vi "9_3_1_2 No_Load_Test_Set 12V for PS1-PS3.vi"(11 "VariantIn":variant caption="Test Config Cluster Variant In") -> (0 "System Error Out":errorcluster, 3 "variantOut":variant caption="Test Config Cluster V ariant Out")   [LabVIEW 2020]
uses:
  <vilib>/Utility/miscctls.llb/LVRowAndColumnTypeDef.ctl
  <userlib>/_ATMF/Tools/Control/__TEST__SEQ__VARIABLES__.ctl
  <userlib>/_ATMF/Tools/Control/__STEP__DATA__.ctl
  <userlib>/_ATMF/Tools/Control/__STEP__DATA__TYPE__.ctl
  <userlib>/_ATMF/Tools/Control/__STEP__DATA__STATUS__TYPE__.ctl
  <userlib>/_ATMF/Tools/Control/__TEST__SEQ__CONFIG__CLUSTER__.ctl
  <userlib>/_ATMF/Control_Typedef/__TEST__STEP__VAR__UI__EXEC__MODE__.ctl
  <vilib>/Utility/miscctls.llb/LVBoundsTypeDef.ctl
  <vilib>/Utility/miscctls.llb/LVPositionTypeDef.ctl
  <userlib>/_ATMF/Tools/Control/__TABLE__ACTION__.ctl
  subvi/DM3058 Function Choose.ctl
  subvi/DCDC_Command.ctl
  70cdd13f-c836-49cb-97c4-706e2b611909.vi
  367b9f9e-7b96-452b-b4ff-c6404e92ffb7.vi
  <vilib>/Utility/file.llb/Write Delimited Spreadsheet (string).vi
  <vilib>/Utility/file.llb/Read Delimited Spreadsheet (string).vi
  <userlib>/_ATMF/Tools/SubVIs/SubPalette_Update_Sequencer_Variable/SEQ.Update_Seq_Var_Module.Action.vi
  <userlib>/_ATMF/Tools/SubVIs/SubPalette_Update_Sequencer_Variable/Set_Max_Min/SEQ.Update_Seq_Var_Module.Set_Max_Min.vi
  <userlib>/_ATMF/Tools/SubVIs/SubPalette_Update_Sequencer_Variable/SEQ.Update_Seq_Var_Module.Numericl_Test.vi
  <userlib>/_ATMF/Tools/SubVIs/SubPalette_Update_Sequencer_Variable/SEQ.Update_Seq_Var_Module.Pass_Fail_Test.vi
  <vilib>/Comparison/Equal/Equal Functor/Equal Functor.lvclass
  <vilib>/addons/_JKI.lib/Serialization/JSON/JKI JSON Serialization.lvlib
panel:
  in  "Instrument Serial":T1
  out "Cell Position":T2
  in  "stepsRing":u16(ring) items=["Next", "End", "--------------", "init", "Power On", "Measure VPS1", "Measure VPS2", "Measure VPS3", "Measure L1 ON", "Measure L3 ON", "Measure UUT D3 ON", "Measure UUT D5 ON", "Measure UUT D6 ON", "Measure UUT D8 ON", "Measure APOS UUT Voltages", "Measure ANEG UUT Voltages", "Measure DPOS UUT Voltages"]
  in  "exitButton":bool
  in  "saveButton":bool
  in  "runButton":bool
  in  "currentRetest":u8
  in  "totalSeqIndex":i32
  in  "currenIndex":i32
  in  "seqData[](Process)":string[][](array[string])
  in  "disMsg":refnum<vi>
  in  "seqData[](Original)":string[][](array[string])
  in  "Tab Control":enum32{"Sequence", "Input", "Output"}(tab)
  in  "stepName":string
  in  "Sequence List":i32[](listbox)=[0]
  in  "seqFilePath":path caption="Sequence File Path :"
  in  "userDef":T3={"VSP1 Min"=13.0, "VSP1 Max"=11.0, "VSP2 Min"=13.0, "VSP3 Max"=11.0, "VSP3 Min"=13.0, "VSP2 Max"=11.0, "L1 Min"=1.164, "L1 Max"=1.236, "L3 Min"=1.164, "L3 Max"=1.236, "APOS Max "=0.5, "ANEG Max"=-0.5, "DPOS Max"=0.5, "D5 Min"=1.164, "D5 Max"=1.236, "D6 Min"=1.164, "D6 Max"=1.236, "D3 Min"=0.873, "D3 Max"=0.927, "D8 Min"=1.164, "D8 Max"=1.236, "APOS Min"=0.5, "ANEG Min"=-0.5, "DPOS Min"=0.5} caption="User Input ( Save by Run Ctrl+R and click \"Save\" button  )"
  in  "varFilePath":path caption="Variable File Path :"
  in  "criteriaINI":path caption="Criteria(.ini) Path :"
  in  "displayMsg":string caption="Display Message"
  in  "testTable":i32(listbox)=-1 caption="Connectivity Test"
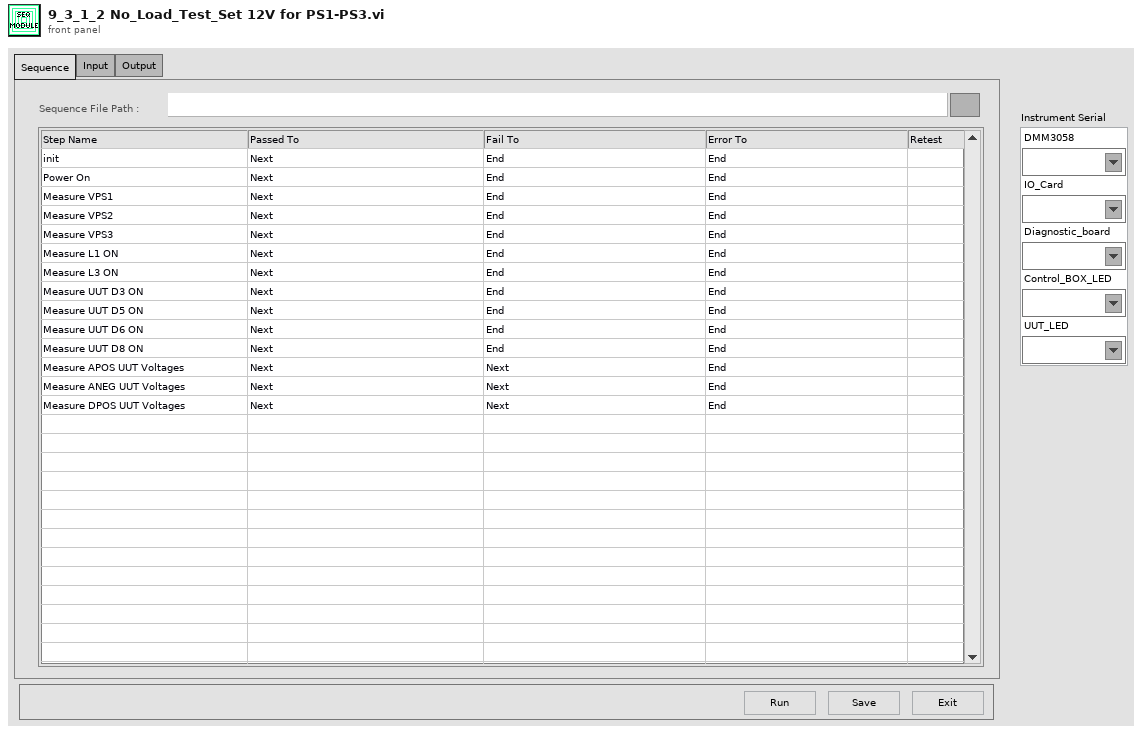
[diagram p1: front panel]
types:
  T1 = cluster{"DMM3058":refnum<visa-resource-name>, "IO_Card":refnum<visa-resource-name>, "Diagnostic_board":refnum<visa-resource-name>, "Control_BOX_LED":refnum<visa-resource-name>, "UUT_LED":refnum<visa-resource-name>}
  T2 = typedef "LVRowAndColumnTypeDef.ctl" = cluster{"Row":i32, "Column":i32}
  T3 = cluster{"VSP1 Min":dbl, "VSP1 Max":dbl, "VSP2 Min":dbl, "VSP3 Max":dbl, "VSP3 Min":dbl, "VSP2 Max":dbl, "L1 Min":dbl, "L1 Max":dbl, "L3 Min":dbl, "L3 Max":dbl, "APOS Max ":dbl, "ANEG Max":dbl, "DPOS Max":dbl, "D5 Min":dbl, "D5 Max":dbl, "D6 Min":dbl, "D6 Max":dbl, "D3 Min":dbl, "D3 Max":dbl, "D8 Min":dbl, "D8 Max":dbl, "APOS Min":dbl, "ANEG Min":dbl, "DPOS Min":dbl}
  T4 = typedef "__TEST__SEQ__VARIABLES__.ctl" = cluster{"stepData":T5, "testConfigCluster":T8}
  T5 = typedef "__STEP__DATA__.ctl" = cluster{"stepType":T6, "stepName":string, "description":string, "min":string, "measure":string, "max":string, "unit":string, "statusType":T7, "runMode":enum16{"Normal", "Skip"}, "viPath":path, "uutError":errorcluster, "passTo":string, "failTo":string, "errorTo":string, "parameter":string, "value":variant, "startTime":timestamp, "intervalLoop":u8, "retest":u8}
  T6 = typedef "__STEP__DATA__TYPE__.ctl" = enum16{"Action", "Pass/Fail Test", "Numeric Limit Test", "String Value Test"}
  T7 = typedef "__STEP__DATA__STATUS__TYPE__.ctl" = enum16{"DONE", "PASS", "FAIL", "ERROR", "SKIPPED"}
  T8 = typedef "__TEST__SEQ__CONFIG__CLUSTER__.ctl" = cluster{"slotIndex":u8, "execMode":T9, "mainConfigFile":path, "criteriaINI":path, "totalResult":bool, "stopIfFail":bool, "userControls":cluster{"dialog":refnum<vi>, "testTable":refnum<vi>, "stopButton":refnum<vi>, "statusBox":refnum<vi>}, "testedResult":enum16{"DONE", "PASS", "FAIL", "ERROR", "SKIPPED"}, "timeStamp":cluster{"Start":timestamp, "End":timestamp}, "repeatNum":u8, "uutInfo":cluster{"s/n":string, "p/n":string, "productRev":string}, "sysLanguage":enum16{"English", "Chinese", "Thai"}, "numOfSocket#":u8, "testRef":string, "testInfo":cluster{"testTime":string, "userID":string, "stationName":string, "testerID":string, "hwVer":string, "swVer":string, "fixtureID":string}}
  T9 = typedef "__TEST__STEP__VAR__UI__EXEC__MODE__.ctl" = enum16{"Run", "Debug", "Edit", "Open VI"}
  T10 = enum16{"open", "replace", "create", "open or create", "replace or create", "replace or create with confirmation"}
  T11 = typedef "LVPositionTypeDef.ctl" = cluster{"Left":i32, "Top":i32}
  T12 = typedef "LVBoundsTypeDef.ctl" = cluster{"Width":u32, "Height":u32}
  T13 = enum32{"Bad", "Idle", "Run top level", "Running"}
  T14 = typedef "__TABLE__ACTION__.ctl" = enum16{"Initial", "Append", "Clear", "Header"}
  T15 = enum16{"StepName", "PassTo", "FailTo", "ErrorTo", "Re-test"}
  T16 = enum16{"StepName", "PassTo", "FailTo", "ErrorTo"}
  T17 = cluster{"Reset (True)":bool, "ID Query (True)":bool, "Auto Range (T:Enable)":bool, "Function (0: DC Volts)":u16, "Range Select":enum16{"200mV", "2V", "20V", "200V", "1000V"}, "Absolute Resolution (0: 5.5 Rate:Slow)":u16}
  T18 = typedef "DM3058 Function Choose.ctl" = enum16{"Close", "Measure", "Config", "Init"}
  T19 = typedef "DCDC_Command.ctl" = enum16{"Reset", "APOS_SENSE", "ANEG_SENSE", "DPOS_SENSE", "FCT_SW1", "FCT_SW2", "FCT_SW3", "ANEG_LOAD", "APOS_LOAD", "DPOS_LOAD", "Short ANEG", "Short APOS", "Short DPOS", "meas_PSU_1_12V", "meas_PSU_2_12V", "meas_PSU_3_12V", "meas_UUT_APOS_voltage", "meas_UUT_ANEG_voltage", "meas_UUT_DPOS_voltage", "meas_LOAD_APOS_voltage", "meas_LOAD_ANEG_voltage", "meas_LOAD_DPOS_voltage", "UUT_FCT_power_SW", "Burn_in_FAN_SW", "FCT_FAN_SW", "FCT_24V_SW", "USB_Reset", "DMM_SW"}
  T20 = typedef "LVPoint32TypeDef.ctl" = cluster{"Horizontal":i32, "Vertical":i32}
  T21 = typedef "LVFontTypeDef.ctl" = cluster{"Font Name":string, "Size":u16, "Bold":bool, "Italic":bool, "Underline":bool, "Strikeout":bool, "Color":u32}
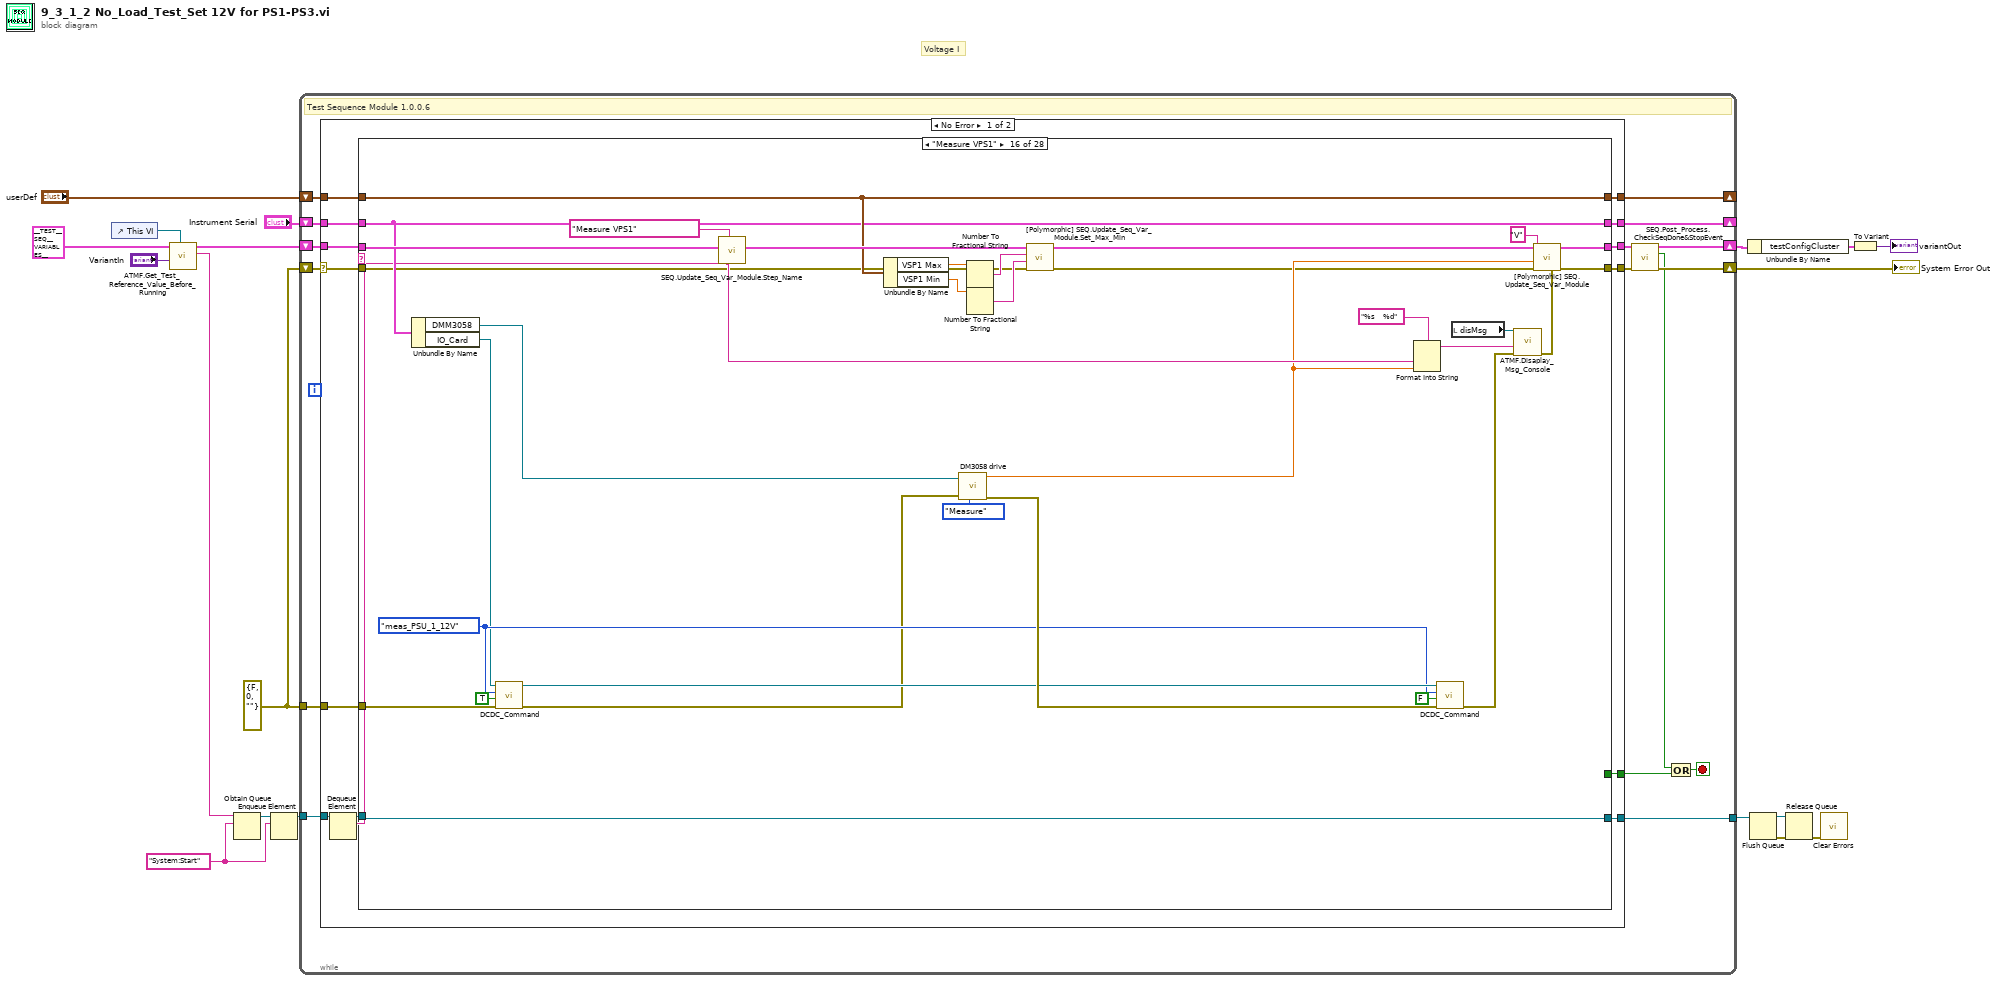
[diagram p0: block diagram]
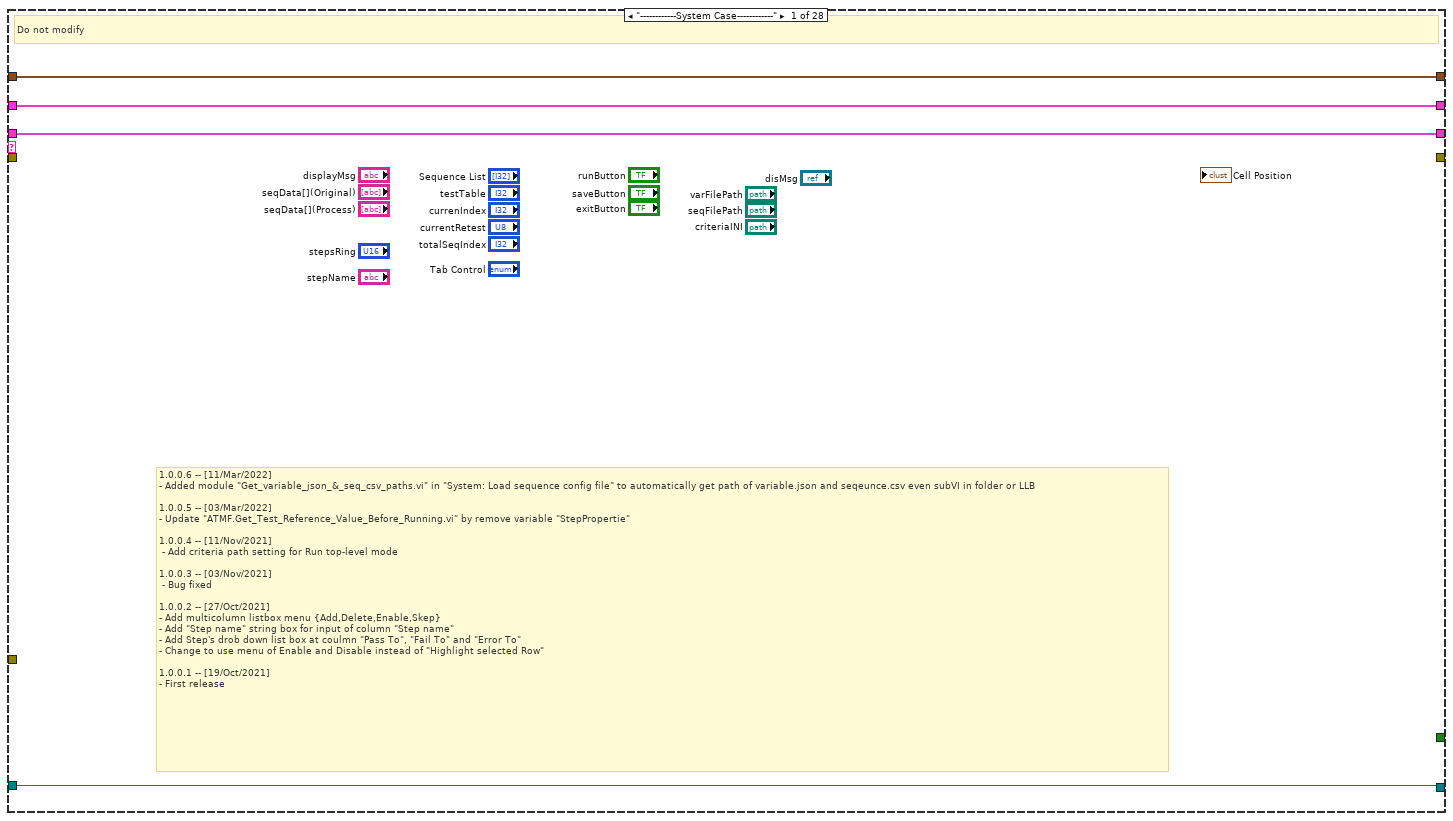
[diagram p2: hidden frame]
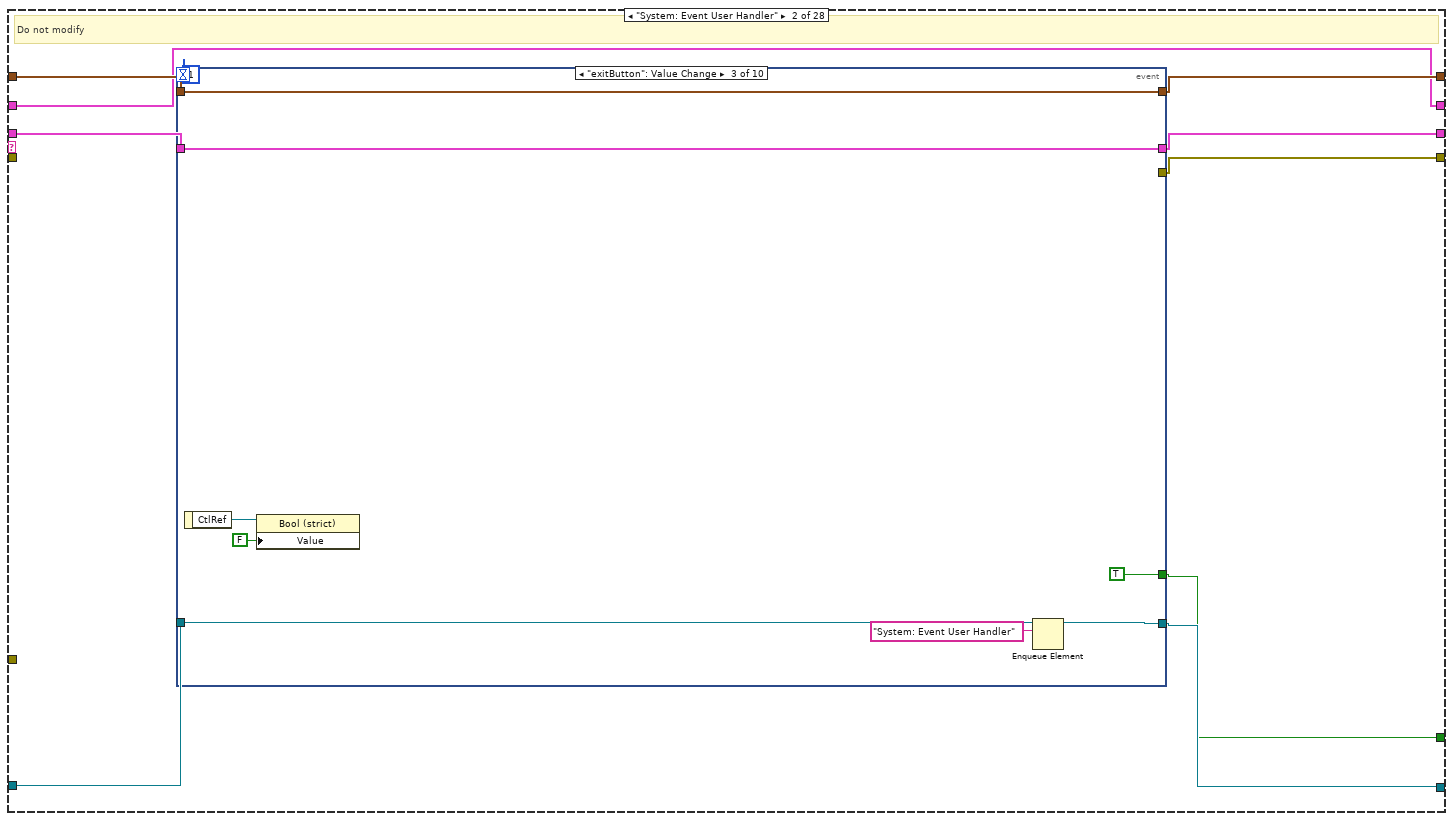
[diagram p3: hidden frame]
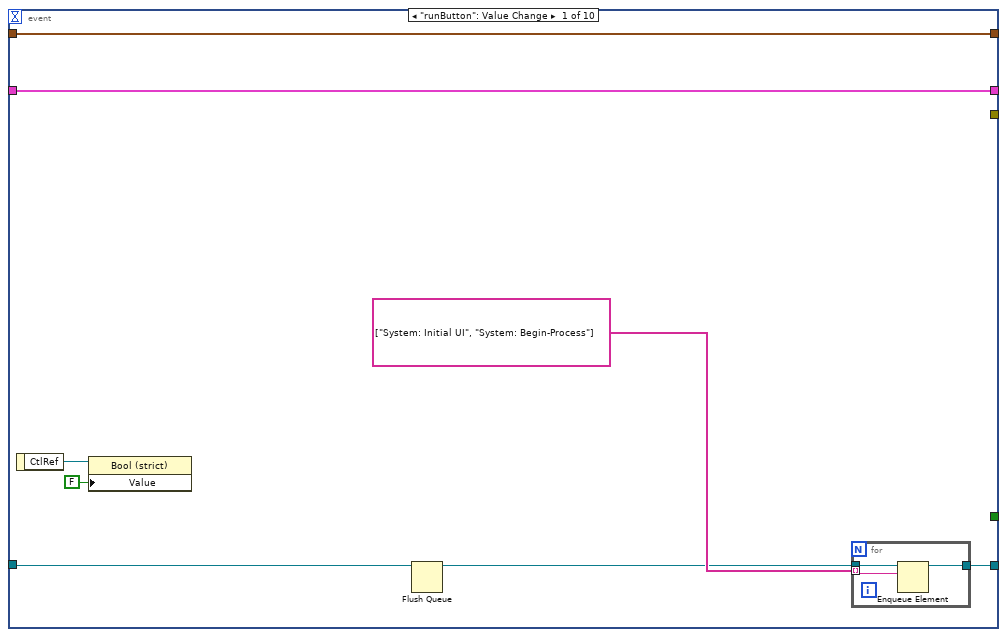
[diagram p4: hidden frame]
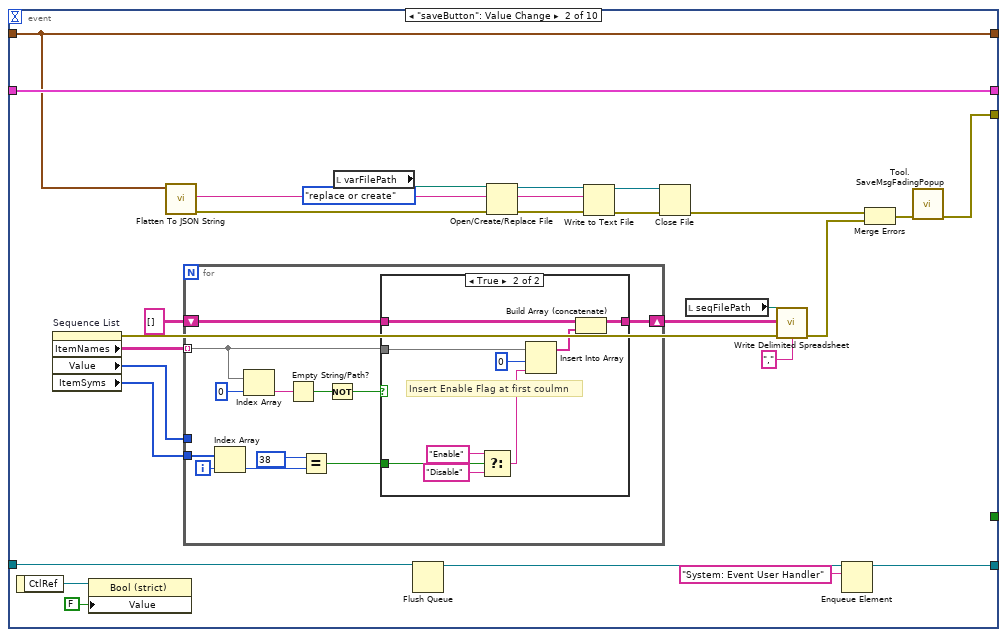
[diagram p5: hidden frame]
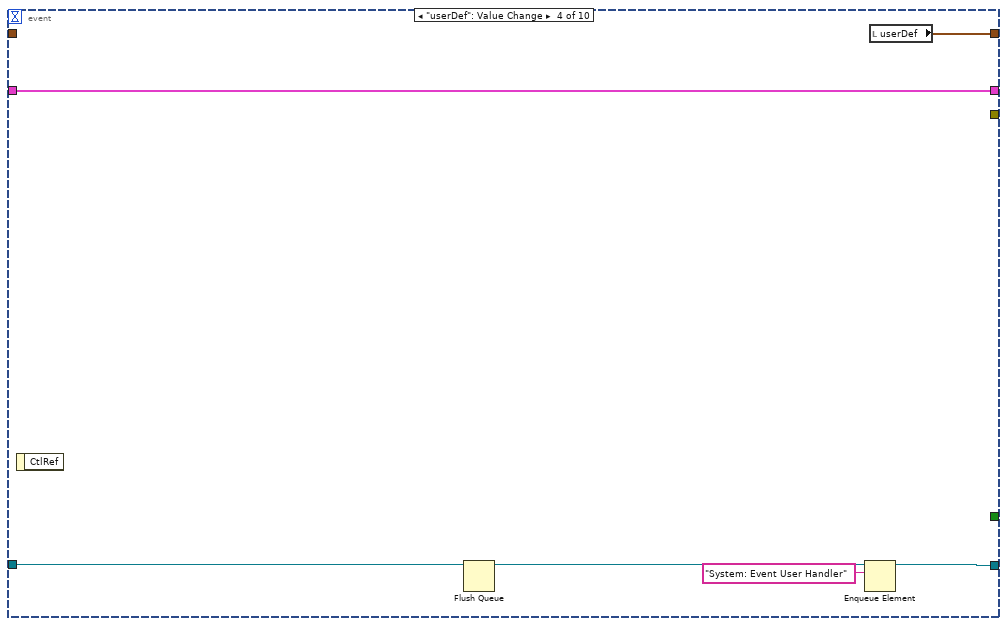
[diagram p7: hidden frame]
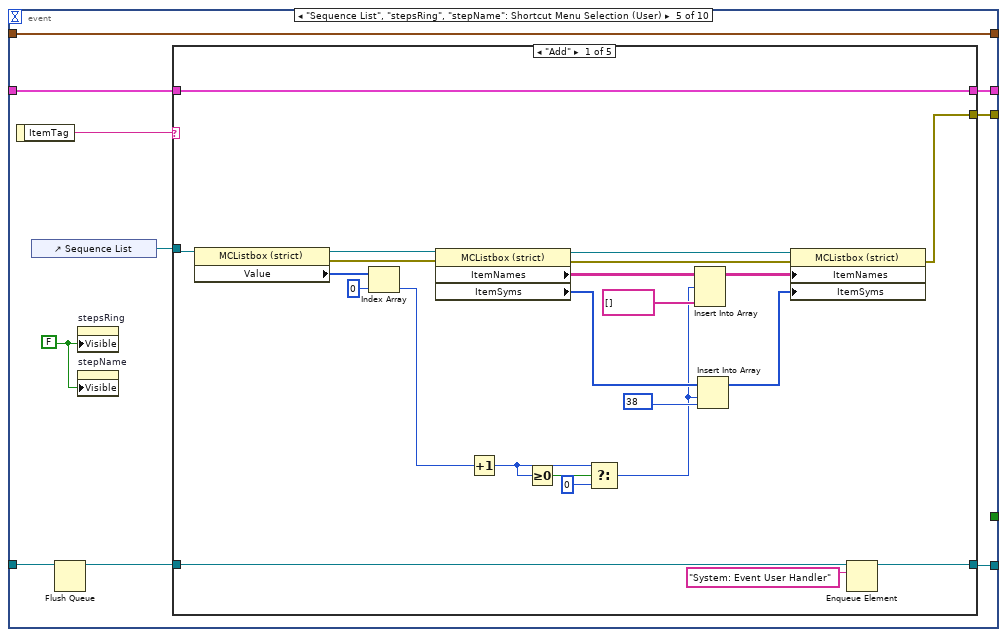
[diagram p8: hidden frame]
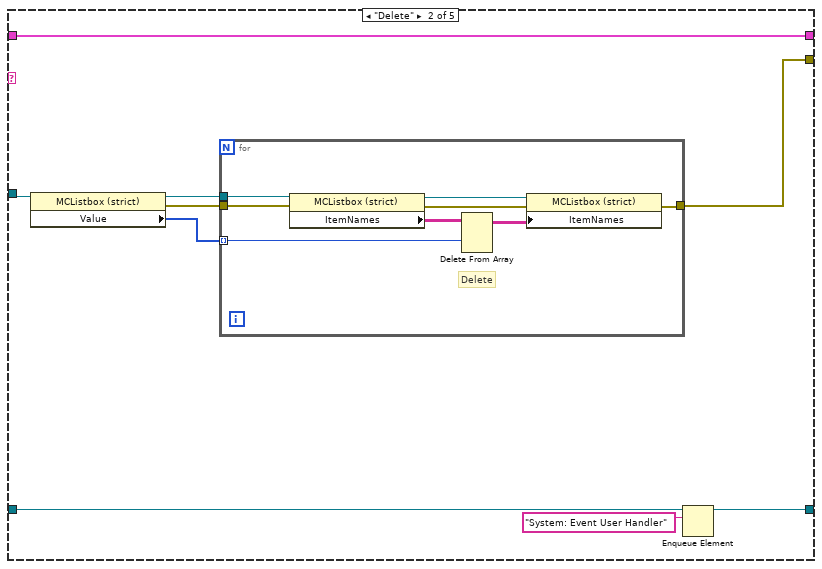
[diagram p9: hidden frame]
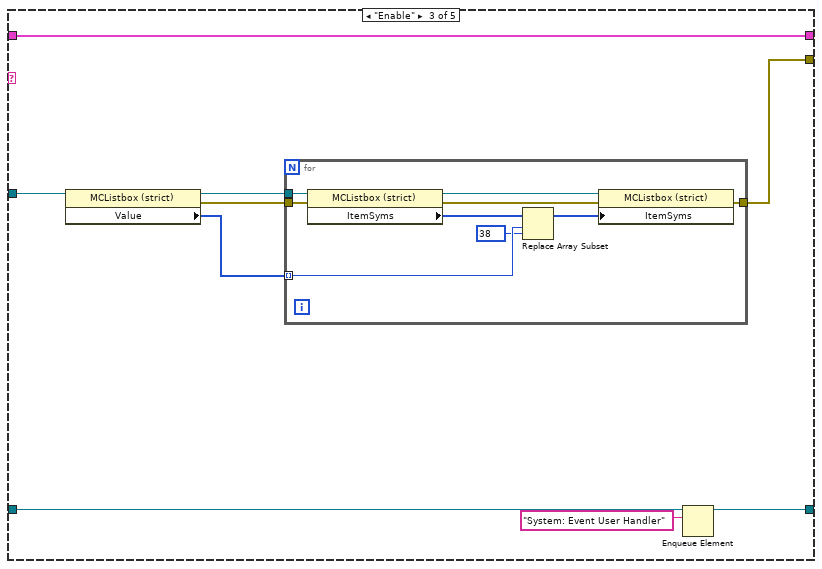
[diagram p10: hidden frame]
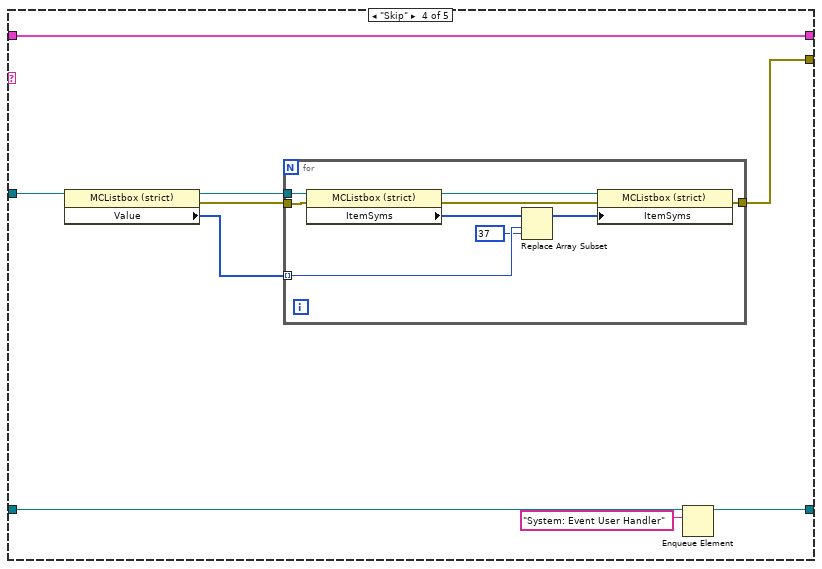
[diagram p11: hidden frame]
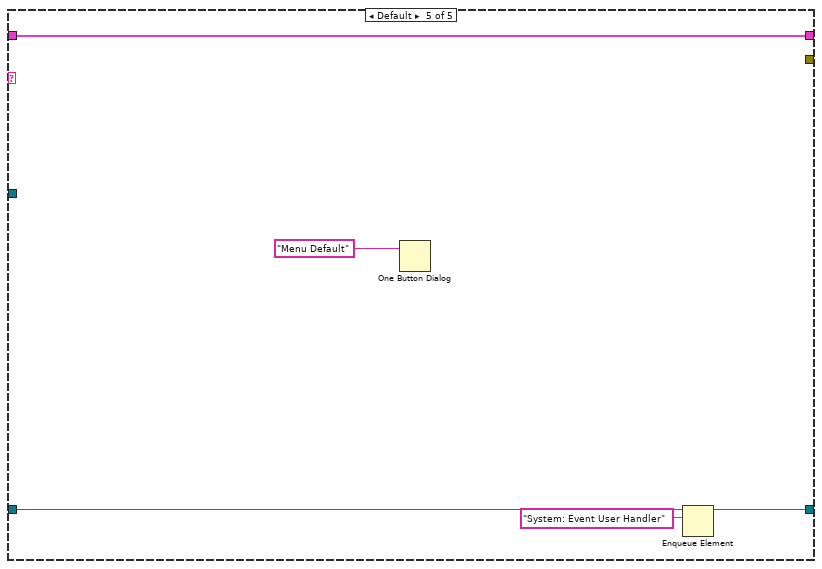
[diagram p12: hidden frame]
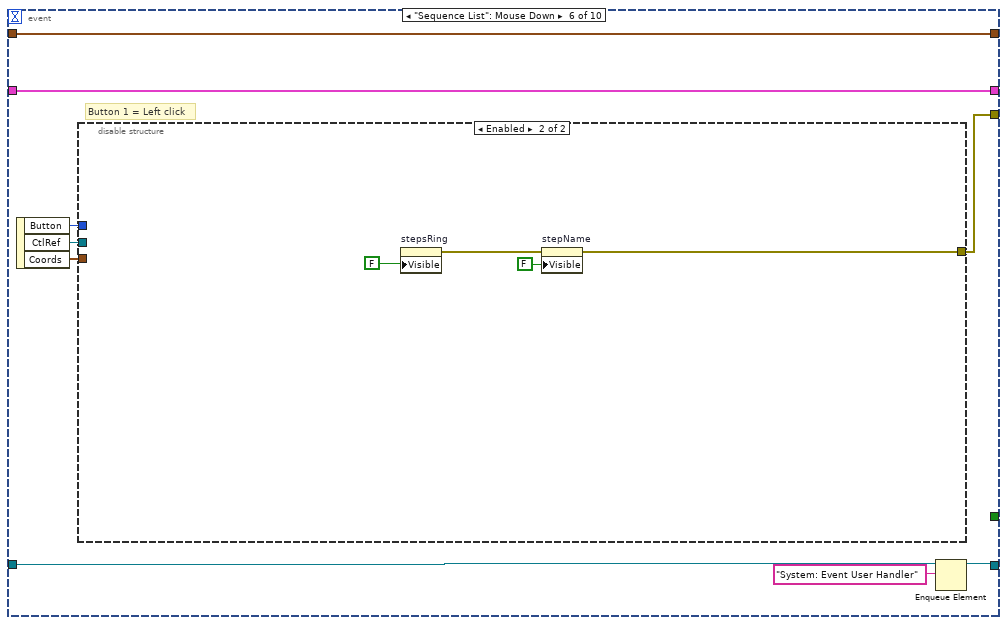
[diagram p13: hidden frame]
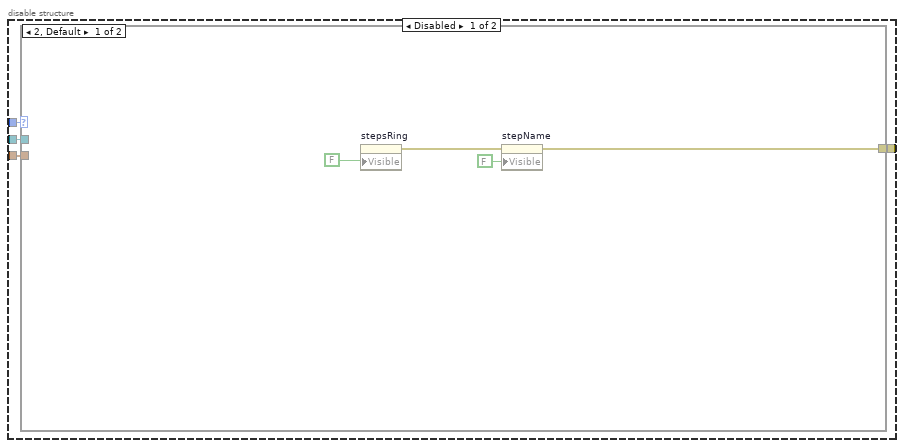
[diagram p14: hidden frame]
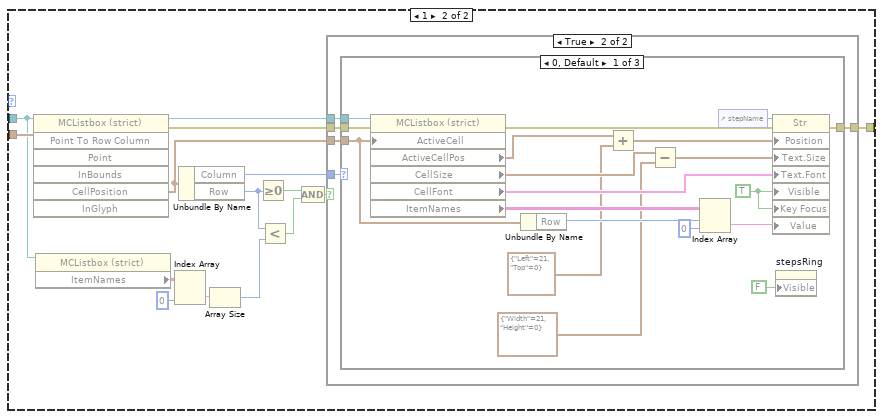
[diagram p15: hidden frame]
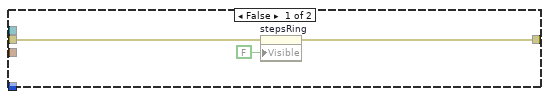
[diagram p16: hidden frame]
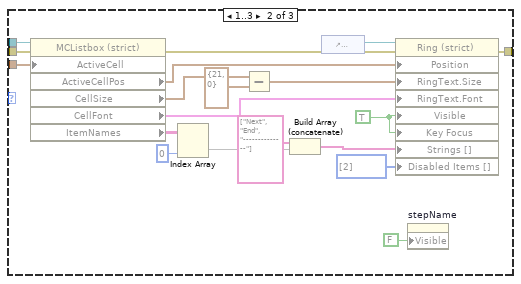
[diagram p17: hidden frame]
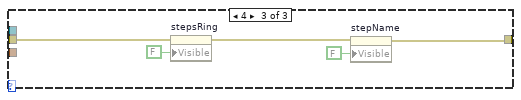
[diagram p18: hidden frame]
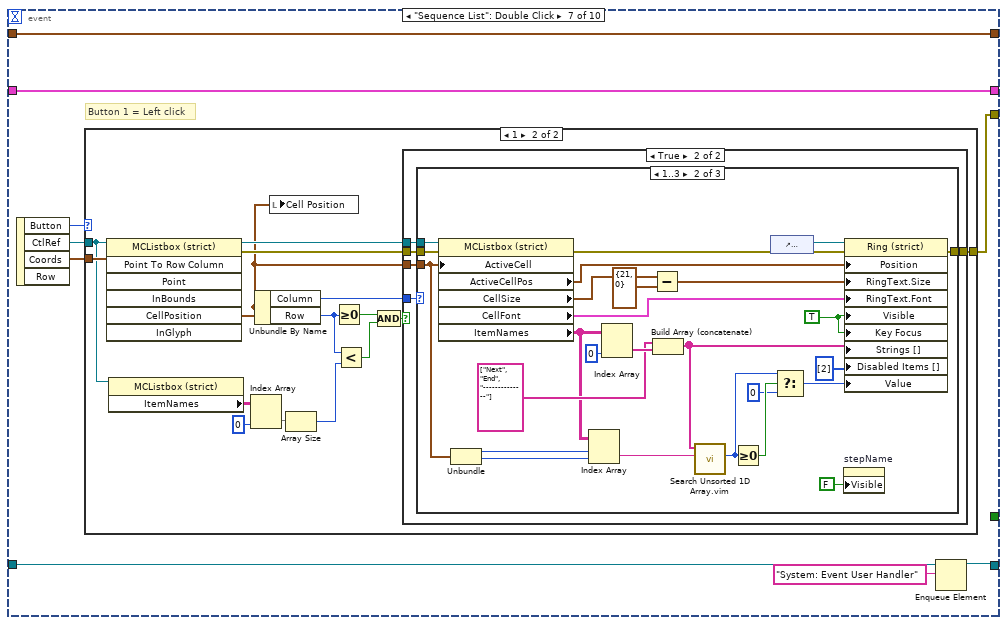
[diagram p19: hidden frame]
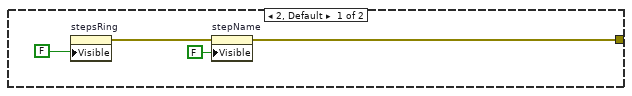
[diagram p20: hidden frame]
diagram:
  w2 = errorcluster {"status"=FALSE, "code"=0, "source"=""} ("UUT Error In")
  w14 = "System:Start"
  # "Voltage I"
  n1 = control-ref of="This VI"() -> (w6:refnum<vi>)
  n2 = call <userlib>:"ATMF.Get_Test_Reference_Value_Before_Running.vi"("viRef"=w6, "Variant"="VariantIn", "seqDataIn"=T4 {"stepData"={"stepType"=enum."Action", "stepName"="", "description"="", "min"="", "measure"="", "max"="", "unit"="", "statusType"=enum."DONE", "runMode"=enum."Normal", "viPath"=path "", "uutError"={"status"=FALSE, "code"=0, "source"=""}, "passTo"="", "failTo"="", "errorTo"="", "parameter"="", "value"=variant(string[][] []), "startTime"=timestamp(0 s since 1904-01-01), "intervalLoop"=1, "retest"=0}, "testConfigCluster"={"slotIndex"=0, "execMode"=enum."Run", "mainConfigFile"=path "", "criteriaINI"=path "", "totalResult"=FALSE, "stopIfFail"=FALSE, "userControls"={"dialog"=refnum, "testTable"=refnum, "stopButton"=refnum, "statusBox"=refnum}, "testedResult"=enum."DONE", "timeStamp"={"Start"=timestamp(0 s since 1904-01-01), "End"=timestamp(0 s since 1904-01-01)}, "repeatNum"=1, "uutInfo"={"s/n"="", "p/n"="", "productRev"=""}, "sysLanguage"=enum."English", "numOfSocket#"=1, "testRef"="", "testInfo"={"testTime"="", "userID"="", "stationName"="", "testerID"="", "hwVer"="", "swVer"="", "fixtureID"=""}}} ("localVar")) -> ("testRef#"=w9:string, "seqDataOut"=w7:T4)  [unwired: 6 in, 1 out]
  n3 = Obtain Queue(name (unnamed)=w9, element data type=w14) -> (queue out=w19:refnum<queue>)  [unwired: 3 in, 2 out]
  n4 = Enqueue Element(queue=w19, element=w14) -> (queue out=w17:refnum<queue>)  [unwired: 2 in, 2 out]
  n5 = while {
    shift-right: [w25] -> w11
    shift-left: w2 -> [w35]
    shift-right: [w27] -> w5
    shift-left: w7 -> [w34]
    tunnel: w17 -> [w33]
    tunnel: [w32] -> w16
    tunnel: w2 -> [w30]
    shift-right: [w29] -> _
    shift-left: "userDef" -> [w31]
    shift-right: [w21] -> _
    shift-left: "Instrument Serial" -> [w20]
    stop <- w22 stop-if-true
    # "Test Sequence Module 1.0.0.6"
    n6 = case shown="No Error" w35 {
      selector: w35 -> [w47 w1245]
      tunnel: [w46 w1245] -> w26
      tunnel: w34 -> [w49 w1252]
      tunnel: [w48 w1252] -> w28
      tunnel: [w45 TRUE] -> w23
      tunnel: [w42 w1250] -> w32
      tunnel: w33 -> [w41 w1247]
      tunnel: w31 -> [w39 w1246]
      tunnel: w30 -> [w40 _]
      tunnel: [w38 w1246] -> w29
      tunnel: [w37 w1244] -> w21
      tunnel: w20 -> [w36 w1244]
      frame No Error {
        n7 = Dequeue Element(queue=w41) -> (queue out=w43:refnum<queue>, element=w44:string)  [unwired: 2 in, 2 out]
        n8 = case shown="\"Measure VPS1\"" w44 {
          selector: w44 -> [_ _ _ _ _ _ _ _ _ _ _ w763 _ w780 w829 w851 w878 w909 w950 w971 w995 w1017 w1040 w1065 w1088 w1141 w1191 w1240]
          tunnel: w49 -> [w52 w60 w438 w472 w484 w535 w622 w638 w683 w707 w740 w767 w770 w812 w842 w874 w906 w938 w961 w984 w1007 w1030 w1053 w1076 w1102 w1154 w1206 w1239]
          tunnel: [w52 w59 w440 w475 w493 w535 w622 w640 w682 w715 w743 w767 w770 w811 w841 w873 w905 w937 w960 w983 w1006 w1029 w1052 w1075 w1099 w1151 w1203 w1234] -> w48
          tunnel: w47 -> [_ _ _ _ _ _ _ _ _ _ _ _ _ w779 w828 w849 w876 w908 w951 w976 w994 w1022 w1045 w1064 w1083 w1140 w1193 _]
          tunnel: [_ w55 _ _ w494 w533 _ _ _ _ _ w759 _ w810 w840 w872 w904 w936 w959 w982 w1005 w1028 w1051 w1074 w1100 w1152 w1204 w1235] -> w46
          tunnel: [_ w56 _ _ _ _ _ _ _ _ w746 TRUE _ _ _ _ _ _ _ _ _ _ _ _ _ _ _ _] -> w45
          tunnel: w43 -> [w51 w63 w450 w473 w491 w536 w628 w642 w681 w714 w742 w765 w769 w809 w839 w871 w903 w935 w958 w981 w1004 w1027 w1050 w1073 w1103 w1155 w1207 w1236]
          tunnel: [w51 w58 w449 w473 w490 w536 w627 w641 w680 w713 w741 w765 w769 w809 w839 w871 w903 w935 w958 w981 w1004 w1027 w1050 w1073 w1103 w1155 w1207 w1236] -> w42
          tunnel: w40 -> [_ _ _ _ _ _ _ _ _ _ _ _ _ w790 w827 w846 w888 w918 w949 w977 w1000 w1023 w1046 w1063 w1096 w1134 w1202 w1237]
          tunnel: w39 -> [w53 w62 w442 w474 w495 w532 w617 w639 w685 w716 w745 w764 w771 w807 w838 w868 w900 w932 w945 w968 w991 w1014 w1037 w1060 w1094 w1147 w1198 w1238]
          tunnel: [w53 w61 w441 w474 w495 w531 w617 w639 w685 w716 w744 w764 w771 w807 w838 w868 w900 w932 w945 w968 w991 w1014 w1037 w1060 w1094 w1147 w1198 w1238] -> w38
          tunnel: [w50 w54 w436 w470 w483 w526 w616 w629 w679 w705 w738 w757 w768 w781 w835 w858 w887 w917 w946 w979 w1002 w1025 w1048 w1071 w1098 w1148 w1200 w1243] -> w37
          tunnel: w36 -> [w50 w54 w436 w470 w483 w526 w616 w629 w679 w705 w738 w757 w768 w806 w835 w858 w887 w917 w946 w979 w1002 w1025 w1048 w1071 w1098 w1148 w1200 w1243]
          frame "------------System Case------------" {
            # "1.0.0.6 -- [11/Mar/2022]\n- Added module \"Get_variable_json_&_seq_csv_paths.vi\" in \"System: Load sequence config file\" to automatically get path of variable.json and seqeunce.csv even subVI in folder or LLB\n\n1.0.0.5 -- [03/Mar/2022]\n- Update \"ATMF.Get_Test_Reference_Value_Before_Running.vi\" by remove variable \"StepPropertie\"\n\n1.0.0.4 -- [11/Nov/2021]\n - Add criteria path setting for Run top-level mode\n\n1.0.0.3 -- [03/Nov/2021]\n - Bug fixed \n\n1.0.0.2 -- [27/Oct/2021]\n- Add multicolumn listbox menu {Add,Delete,Enable,Skep}\n- Add \"Step name\" string box for input of column \"Step name\"\n- Add Step's drob down list box at coulmn \"Pass To\", \"Fail To\" and \"Error To\"\n- Change to use menu of Enable and Disable instead of \"Highlight selected Row\"\n\n1.0.0.1 -- [19/Oct/2021]\n- First release"
            # "Do not modify"
          }
          frame "System: Event User Handler" {
            # "Do not modify"
            n9 = event shown="[2] \"exitButton\": Value Change" {
              selector: _ -> [_ _ _ _ _ _ _ _ _ _]
              dyn-events: _ -> [_ _ _ _ _ _ _ _ _ _]
              timeout: -1 -> [_ _ _ _ _ _ _ _ _ _]
              tunnel: w63 -> [w64 w86 w126 w133 w142 w236 w323 w404 w424 w433]
              tunnel: w62 -> [w71 w99 w132 _ w147 w238 w325 w415 w432 w435]
              tunnel: [w71 w99 w132 w135 w147 w238 w325 w415 w432 w435] -> w61
              tunnel: w60 -> [w70 w102 w131 w138 w145 w237 w324 w414 w431 w434]
              tunnel: [w70 w102 w131 w138 w146 w237 w324 w414 w431 w434] -> w59
              tunnel: [w69 w89 w127 w137 w148 w235 w322 w405 w425 w433] -> w58
              tunnel: [_ _ TRUE _ _ _ _ _ _ _] -> w56
              tunnel: [_ w97 _ _ w141 w231 w318 w411 w428 _] -> w55
              event "runButton": Value Change {
                n10 = event-data() -> ("CtlRef"=w68:refnum<vi>)  [unwired: 1 in]
                n11 = property class="Bool (strict)"(reference=w68, "Value"=FALSE) -> ()  [unwired: 1 in, 2 out]
                n12 = Flush Queue(queue=w64) -> (queue out=w65:refnum<queue>)  [unwired: 1 in, 2 out]
                n13 = for {
                  tunnel: w65 -> [w74]
                  tunnel: [w73] -> w69
                  tunnel: string[] ["System: Initial UI", "System: Begin-Process"] -> [w72] mode=indexing
                  n14 = Enqueue Element(queue=w74, element=w72) -> (queue out=w73:refnum<queue>)  [unwired: 2 in, 2 out]
                }
              }
              event "saveButton": Value Change {
                n15 = event-data() -> ("CtlRef"=w101:refnum<vi>)  [unwired: 1 in]
                n16 = property on="Sequence List" class="MCListbox (strict)"() -> (error out=w85:errorcluster, "ItemNames"=w81:string[][], "Value"=w82:i32[], "ItemSyms"=w75:i32[])  [unwired: 2 in, 1 out]
                n17 = property class="Bool (strict)"(reference=w101, "Value"=FALSE) -> ()  [unwired: 1 in, 2 out]
                n18 = call <vilib>:"Flatten To JSON String.vi"("Variant"=w99) -> ("error out"=w98:errorcluster, "JSON String"=w91:string)  [unwired: 9 in]
                n19 = for {
                  tunnel: w82 -> [_]
                  tunnel: w81 -> [w112] mode=indexing
                  shift-right: [w108] -> w79
                  shift-left: string[][] [] -> [w109]
                  tunnel: w75 -> [w107]
                  i -> [w106]
                  n20 = Index Array(array=w107, index=w106) -> (element=w105:i32)
                  n21 = Index Array(array=w112, index=0) -> (element=w110:string)
                  n22 = Empty String/Path?(string/path=w110) -> (empty?=w114:bool)
                  n23 = Equal?(x=38, y=w105) -> (x = y?=w103:bool)
                  n24 = Not(x=w114) -> (.not. x?=w113:bool)
                  n25 = case shown="True" w113 {
                    tunnel: w112 -> [_ w124]
                    tunnel: w109 -> [w115 w120]
                    tunnel: [w115 w119] -> w108
                    tunnel: w103 -> [_ w116]
                    frame False {
                    }
                    frame True {
                      # "Insert Enable Flag at first coulmn"
                      n26 = Select(t="Enable", s=w116, f="Disable") -> (s? t:f=w121:string)
                      n27 = Insert Into Array(array=w124, index=0, new element=w121) -> (w118:string[])
                      n28 = Build Array (concatenate)(w120, w118) -> (w119:string[][])
                    }
                  }
                }
                n29 = local read "varFilePath"() -> (w92:path)
                n30 = Flush Queue(queue=w86) -> (queue out=w87:refnum<queue>)  [unwired: 1 in, 2 out]
                n31 = Open/Create/Replace File(file path (use dialog)=w92, error in=w98, operation (0:open)=T10."replace or create") -> (refnum out=w94:refnum<file>, error out=w96:errorcluster)  [unwired: 3 in, 1 out]
                n32 = Write to Text File(file (use dialog)=w94, text=w91, error in=w96) -> (refnum out=w93:refnum<file>, error out=w95:errorcluster)  [unwired: 1 in, 1 out]
                n33 = Close File(refnum=w93, error in=w95) -> (error out=w77:errorcluster)  [unwired: 1 out]
                n34 = local read "seqFilePath"() -> (w83:path)
                n35 = call-poly <vilib>:"Write Delimited Spreadsheet.vi"("file path (dialog if empty)"=w83, "2D data"=w79, "error in (no error)"=w85, "delimiter (\\t)"="," ("delimiter (\\t)")) -> ("error out"=w78:errorcluster)  [unwired: 10 in, 1 out]
                n36 = Enqueue Element(queue=w87, element="System: Event User Handler") -> (queue out=w89:refnum<queue>)  [unwired: 2 in, 2 out]
                n37 = Merge Errors(w77, w78) -> (w76:errorcluster)
                n38 = call <userlib>:"Tool.SaveMsgFadingPopup.vi"("error in"=w76) -> ("error out"=w97:errorcluster)  [unwired: 10 in]
              }
              event "exitButton": Value Change {
                n39 = event-data() -> ("CtlRef"=w130:refnum<vi>)  [unwired: 1 in]
                n40 = property class="Bool (strict)"(reference=w130, "Value"=FALSE) -> ()  [unwired: 1 in, 2 out]
                n41 = Enqueue Element(queue=w126, element="System: Event User Handler") -> (queue out=w127:refnum<queue>)  [unwired: 2 in, 2 out]
              }
              event "userDef": Value Change {
                n42 = event-data() -> ()  [unwired: 1 in, 1 out]
                n43 = Flush Queue(queue=w133) -> (queue out=w134:refnum<queue>)  [unwired: 1 in, 2 out]
                n44 = Enqueue Element(queue=w134, element="System: Event User Handler") -> (queue out=w137:refnum<queue>)  [unwired: 2 in, 2 out]
                n45 = local read "userDef"() -> (w135:T3)
              }
              event "Sequence List", "stepsRing", "stepName": Shortcut Menu Selection (User) {
                w139 = FALSE
                n46 = event-data() -> ("ItemTag"=w144:string)  [unwired: 1 in]
                n47 = control-ref of="Sequence List"() -> (w140:refnum<vi>)
                n48 = Flush Queue(queue=w142) -> (queue out=w143:refnum<queue>)  [unwired: 1 in, 2 out]
                n49 = property on="stepsRing" class="Ring (strict)"("Visible"=w139) -> ()  [unwired: 2 in, 2 out]
                n50 = property on="stepName" class="Str"("Visible"=w139) -> ()  [unwired: 2 in, 2 out]
                n51 = case shown="\"Add\"" w144 {
                  tunnel: [w171 w180 w197 w215 w229] -> w148
                  tunnel: w143 -> [w169 w178 w195 w213 w227]
                  tunnel: [w168 w177 w194 w212 w226] -> w146
                  tunnel: w145 -> [w168 w177 w194 w212 w226]
                  tunnel: w140 -> [w149 w173 w193 w211 _]
                  tunnel: [w161 w174 w189 w207 _] -> w141
                  frame "Add" {
                    n52 = property class="MCListbox (strict)"(reference=w149) -> (reference out=w165:refnum<vi>, error out=w164:errorcluster, "Value"=w167:i32[])  [unwired: 1 in]
                    n53 = Index Array(array=w167, index=0) -> (element=w152:i32)
                    n54 = property class="MCListbox (strict)"(reference=w165, error in=w164) -> (reference out=w163:refnum<vi>, error out=w162:errorcluster, "ItemNames"=w160:string[][], "ItemSyms"=w157:i32[])
                    n55 = Increment(x=w152) -> (x+1=w154:i32)
                    n56 = Greater Or Equal To 0?(x=w154) -> (x >= 0?=w153:bool)
                    n57 = Select(t=w154, s=w153, f=0) -> (s? t:f=w151:i32)
                    n58 = Insert Into Array(array=w160, index (row)=w151, new element=string[] [] ("new element/subarray")) -> (w159:string[][])  [unwired: 1 in]
                    n59 = Insert Into Array(array=w157, index=w151, new element=38) -> (w155:i32[])
                    n60 = property class="MCListbox (strict)"(reference=w163, error in=w162, "ItemNames"=w159, "ItemSyms"=w155) -> (error out=w161:errorcluster)  [unwired: 1 out]
                    n61 = Enqueue Element(queue=w169, element="System: Event User Handler") -> (queue out=w171:refnum<queue>)  [unwired: 2 in, 2 out]
                  }
                  frame "Delete" {
                    n62 = property class="MCListbox (strict)"(reference=w173) -> (reference out=w176:refnum<vi>, error out=w175:errorcluster, "Value"=w172:i32[])  [unwired: 1 in]
                    n63 = for {
                      tunnel: w176 -> [w188]
                      tunnel: w175 -> [w187]
                      tunnel: [w184] -> w174
                      tunnel: w172 -> [w182] mode=indexing
                      # "Delete"
                      n64 = property class="MCListbox (strict)"(reference=w188, error in=w187) -> (reference out=w186:refnum<vi>, error out=w185:errorcluster, "ItemNames"=w183:string[][])
                      n65 = Delete From Array(array=w183, index (row)=w182) -> (array with subset deleted=w181:string[][])  [unwired: 2 in, 1 out]
                      n66 = property class="MCListbox (strict)"(reference=w186, error in=w185, "ItemNames"=w181) -> (error out=w184:errorcluster)  [unwired: 1 out]
                    }
                    n67 = Enqueue Element(queue=w178, element="System: Event User Handler") -> (queue out=w180:refnum<queue>)  [unwired: 2 in, 2 out]
                  }
                  frame "Enable" {
                    n68 = property class="MCListbox (strict)"(reference=w193) -> (reference out=w191:refnum<vi>, error out=w190:errorcluster, "Value"=w192:i32[])  [unwired: 1 in]
                    n69 = for {
                      tunnel: w192 -> [w202] mode=indexing
                      tunnel: w191 -> [w206]
                      tunnel: w190 -> [w200]
                      tunnel: [w198] -> w189
                      n70 = property class="MCListbox (strict)"(reference=w206, error in=w200) -> (reference out=w204:refnum<vi>, error out=w199:errorcluster, "ItemSyms"=w205:i32[])
                      n71 = Replace Array Subset(array=w205, new element=38, index=w202) -> (w203:i32[])
                      n72 = property class="MCListbox (strict)"(reference=w204, error in=w199, "ItemSyms"=w203) -> (error out=w198:errorcluster)  [unwired: 1 out]
                    }
                    n73 = Enqueue Element(queue=w195, element="System: Event User Handler") -> (queue out=w197:refnum<queue>)  [unwired: 2 in, 2 out]
                  }
                  frame "Skip" {
                    n74 = property class="MCListbox (strict)"(reference=w211) -> (reference out=w209:refnum<vi>, error out=w208:errorcluster, "Value"=w210:i32[])  [unwired: 1 in]
                    n75 = for {
                      tunnel: w210 -> [w220] mode=indexing
                      tunnel: w209 -> [w224]
                      tunnel: w208 -> [w218]
                      tunnel: [w216] -> w207
                      n76 = property class="MCListbox (strict)"(reference=w224, error in=w218) -> (reference out=w222:refnum<vi>, error out=w217:errorcluster, "ItemSyms"=w223:i32[])
                      n77 = Replace Array Subset(array=w223, new element=37, index=w220) -> (w221:i32[])
                      n78 = property class="MCListbox (strict)"(reference=w222, error in=w217, "ItemSyms"=w221) -> (error out=w216:errorcluster)  [unwired: 1 out]
                    }
                    n79 = Enqueue Element(queue=w213, element="System: Event User Handler") -> (queue out=w215:refnum<queue>)  [unwired: 2 in, 2 out]
                  }
                  frame Default {
                    n80 = One Button Dialog(message="Menu Default") -> ()  [unwired: 1 in, 1 out]
                    n81 = Enqueue Element(queue=w227, element="System: Event User Handler") -> (queue out=w229:refnum<queue>)  [unwired: 2 in, 2 out]
                  }
                }
              }
              event "Sequence List": Mouse Down {
                # "Button 1 = Left click"
                n82 = event-data() -> ("Button"=w230:u16, "CtlRef"=w232:refnum<vi>, "Coords"=w233:T20)  [unwired: 1 in]
                n83 = disable-structure shown="Enabled" {
                  disable-tunnel: w233 -> [w242 _]
                  disable-tunnel: w232 -> [w241 _]
                  disable-tunnel: [w240 w313] -> w231
                  disable-tunnel: w230 -> [w239 _]
                  frame Disabled {
                    n84 = case shown="2, Default" w239 {
                      tunnel: w242 -> [_ w261]
                      tunnel: w241 -> [_ w257]
                      tunnel: [w243 w247] -> w240
                      frame 2, Default {
                        n85 = property on="stepsRing" class="Ring (strict)"("Visible"=FALSE) -> (error out=w245:errorcluster)  [unwired: 2 in, 1 out]
                        n86 = property on="stepName" class="Str"(error in=w245, "Visible"=FALSE) -> (error out=w243:errorcluster)  [unwired: 1 in, 1 out]
                      }
                      frame 1 {
                        n87 = invoke class="MCListbox (strict)" method="Point To Row Column"(reference=w257, "Point"=w261) -> (reference out=w260:refnum<vi>, error out=w259:errorcluster, "CellPosition"=w258:T2)  [unwired: 5 in, 4 out]
                        n88 = property class="MCListbox (strict)"(reference=w257) -> ("ItemNames"=w256:string[][])  [unwired: 1 in, 2 out]
                        n89 = Index Array(array=w256, index (col)=0 ("disabled index (col)")) -> (element=w254:string[])  [unwired: 1 in]
                        n90 = Unbundle By Name(w258) -> ("Column"=w248:i32, "Row"=w251:i32)
                        n91 = Array Size(array=w254) -> (size(s)=w250:i32)
                        n92 = Greater Or Equal To 0?(x=w251) -> (x >= 0?=w253:bool)
                        n93 = Less?(x=w251, y=w250) -> (x < y?=w249:bool)
                        n94 = Compound Arithmetic op=AND(w253, w249) -> (w252:bool)
                        n95 = case shown="True" w252 {
                          tunnel: w260 -> [_ w269]
                          tunnel: w259 -> [w264 w268]
                          tunnel: w258 -> [_ w267]
                          tunnel: [w263 w266] -> w247
                          tunnel: w248 -> [_ w265]
                          frame False {
                            n96 = property on="stepsRing" class="Ring (strict)"(error in=w264, "Visible"=FALSE) -> (error out=w263:errorcluster)  [unwired: 1 in, 1 out]
                          }
                          frame True {
                            n97 = case shown="0, Default" w265 {
                              tunnel: w269 -> [w286 w307 _]
                              tunnel: w268 -> [w284 w306 w311]
                              tunnel: w267 -> [w281 w305 _]
                              tunnel: [w287 w291 w308] -> w266
                              frame 0, Default {
                                w276 = TRUE ("Visible")
                                n98 = property on="Property Node" class="MCListbox (strict)"(reference=w286, error in=w284, "ActiveCell"=w281) -> (error out=w285:errorcluster, "ActiveCellPos"=w272:T11, "CellSize"=w275:T12, "CellFont"=w283:T21, "ItemNames"=w282:string[][])  [unwired: 1 out]
                                n99 = Unbundle By Name(w281) -> ("Row"=w280:i32)
                                n100 = Add(x=w272, y=T11 {"Left"=21, "Top"=0}) -> (x+y=w271:T11)
                                n101 = Subtract(x=w275, y=T12 {"Width"=21, "Height"=0}) -> (x-y=w273:T12)
                                n102 = Index Array(array=w282, index (row)=w280, index (col)=0 ("disabled index (col)")) -> (element=w278:string)
                                n103 = control-ref of="stepName"() -> (w288:refnum<vi>)
                                n104 = property on="Property Node" class="Str"(reference=w288, error in=w285, "Position"=w271, "Text.Size"=w273, "Text.Font"=w283, "Visible"=w276, "Key Focus"=w276, "Value"=w278) -> (error out=w287:errorcluster)  [unwired: 1 out]
                                n105 = property on="stepsRing" class="Ring (strict)"("Visible"=FALSE) -> ()  [unwired: 2 in, 2 out]
                              }
                              frame 1..3 {
                                w297 = TRUE ("Visible")
                                n106 = property on="Property Node" class="MCListbox (strict)"(reference=w307, error in=w306, "ActiveCell"=w305) -> (error out=w304:errorcluster, "ActiveCellPos"=w302:T11, "CellSize"=w300:T12, "CellFont"=w301:T21, "ItemNames"=w296:string[][])  [unwired: 1 out]
                                n107 = Index Array(array=w296, index (col)=0 ("disabled index (col)")) -> (element=w294:string[])  [unwired: 1 in]
                                n108 = Subtract(x=w300, y=T12 {"Width"=21, "Height"=0} ("x")) -> (x-y=w299:T12)
                                n109 = Build Array (concatenate)(string[] ["Next", "End", "--------------"], w294) -> (w292:string[])
                                n110 = control-ref of="stepsRing"() -> (w303:refnum<vi>)
                                n111 = property on="Property Node" class="Ring (strict)"(reference=w303, error in=w304, "Position"=w302, "RingText.Size"=w299, "RingText.Font"=w301, "Visible"=w297, "Key Focus"=w297, "Strings []"=w292, "Disabled Items []"=i32[] [2]) -> (error out=w291:errorcluster)  [unwired: 1 out]
                                n112 = property on="stepName" class="Str"("Visible"=FALSE) -> ()  [unwired: 2 in, 2 out]
                              }
                              frame 4 {
                                n113 = property on="stepsRing" class="Ring (strict)"(error in=w311, "Visible"=FALSE) -> (error out=w309:errorcluster)  [unwired: 1 in, 1 out]
                                n114 = property on="stepName" class="Str"(error in=w309, "Visible"=FALSE) -> (error out=w308:errorcluster)  [unwired: 1 in, 1 out]
                              }
                            }
                          }
                        }
                      }
                    }
                  }
                  frame Enabled {
                    n115 = property on="stepsRing" class="Ring (strict)"("Visible"=FALSE) -> (error out=w316:errorcluster)  [unwired: 2 in, 1 out]
                    n116 = property on="stepName" class="Str"(error in=w316, "Visible"=FALSE) -> (error out=w313:errorcluster)  [unwired: 1 in, 1 out]
                  }
                }
                n117 = Enqueue Element(queue=w236, element="System: Event User Handler") -> (queue out=w235:refnum<queue>)  [unwired: 2 in, 2 out]
              }
              event "Sequence List": Double Click {
                # "Button 1 = Left click"
                n118 = event-data() -> ("Button"=w317:u16, "CtlRef"=w319:refnum<vi>, "Coords"=w320:T20)  [unwired: 1 in, 1 out]
                n119 = case shown="1" w317 {
                  tunnel: w320 -> [_ w344]
                  tunnel: w319 -> [_ w341]
                  tunnel: [w326 w331] -> w318
                  frame 2, Default {
                    n120 = property on="stepsRing" class="Ring (strict)"("Visible"=FALSE) -> (error out=w328:errorcluster)  [unwired: 2 in, 1 out]
                    n121 = property on="stepName" class="Str"(error in=w328, "Visible"=FALSE) -> (error out=w326:errorcluster)  [unwired: 1 in, 1 out]
                  }
                  frame 1 {
                    n122 = invoke class="MCListbox (strict)" method="Point To Row Column"(reference=w341, "Point"=w344) -> (reference out=w343:refnum<vi>, error out=w342:errorcluster, "CellPosition"=w330:T2)  [unwired: 5 in, 4 out]
                    n123 = property class="MCListbox (strict)"(reference=w341) -> ("ItemNames"=w340:string[][])  [unwired: 1 in, 2 out]
                    n124 = Index Array(array=w340, index (col)=0 ("disabled index (col)")) -> (element=w338:string[])  [unwired: 1 in]
                    n125 = Unbundle By Name(w330) -> ("Column"=w332:i32, "Row"=w335:i32)
                    n126 = local write "Cell Position"(w330) -> ()
                    n127 = Array Size(array=w338) -> (size(s)=w334:i32)
                    n128 = Greater Or Equal To 0?(x=w335) -> (x >= 0?=w337:bool)
                    n129 = Less?(x=w335, y=w334) -> (x < y?=w333:bool)
                    n130 = Compound Arithmetic op=AND(w337, w333) -> (w336:bool)
                    n131 = case shown="True" w336 {
                      tunnel: w343 -> [_ w352]
                      tunnel: w342 -> [w347 w351]
                      tunnel: w330 -> [_ w350]
                      tunnel: [w346 w349] -> w331
                      tunnel: w332 -> [_ w348]
                      frame False {
                        n132 = property on="stepsRing" class="Ring (strict)"(error in=w347, "Visible"=FALSE) -> (error out=w346:errorcluster)  [unwired: 1 in, 1 out]
                      }
                      frame True {
                        n133 = case shown="1..3" w348 {
                          tunnel: w352 -> [w369 w397 _]
                          tunnel: w351 -> [w367 w396 w401]
                          tunnel: w350 -> [w364 w380 _]
                          tunnel: [w370 w384 w398] -> w349
                          frame 0, Default {
                            w359 = TRUE ("Visible")
                            n134 = property on="Property Node" class="MCListbox (strict)"(reference=w369, error in=w367, "ActiveCell"=w364) -> (error out=w368:errorcluster, "ActiveCellPos"=w355:T11, "CellSize"=w358:T12, "CellFont"=w366:T21, "ItemNames"=w365:string[][])  [unwired: 1 out]
                            n135 = Unbundle By Name(w364) -> ("Row"=w363:i32)
                            n136 = Add(x=w355, y=T11 {"Left"=21, "Top"=0}) -> (x+y=w354:T11)
                            n137 = Subtract(x=w358, y=T12 {"Width"=21, "Height"=0}) -> (x-y=w356:T12)
                            n138 = Index Array(array=w365, index (row)=w363, index (col)=0 ("disabled index (col)")) -> (element=w361:string)
                            n139 = control-ref of="stepName"() -> (w371:refnum<vi>)
                            n140 = property on="Property Node" class="Str"(reference=w371, error in=w368, "Position"=w354, "Text.Size"=w356, "Text.Font"=w366, "Visible"=w359, "Key Focus"=w359, "Value"=w361) -> (error out=w370:errorcluster)  [unwired: 1 out]
                            n141 = property on="stepsRing" class="Ring (strict)"("Visible"=FALSE) -> ()  [unwired: 2 in, 2 out]
                          }
                          frame 1..3 {
                            w388 = TRUE ("Visible")
                            n142 = property on="Property Node" class="MCListbox (strict)"(reference=w397, error in=w396, "ActiveCell"=w380) -> (error out=w395:errorcluster, "ActiveCellPos"=w393:T11, "CellSize"=w391:T12, "CellFont"=w392:T21, "ItemNames"=w381:string[][])  [unwired: 1 out]
                            n143 = Unbundle(w380) -> ("Row"=w379:i32, "Column"=w378:i32)
                            n144 = Index Array(array=w381, index (row)=w379, index (col)=w378) -> (element=w376:string)
                            n145 = Index Array(array=w381, index (col)=0 ("disabled index (col)")) -> (element=w386:string[])  [unwired: 1 in]
                            n146 = Subtract(x=w391, y=T12 {"Width"=21, "Height"=0} ("x")) -> (x-y=w390:T12)
                            n147 = Build Array (concatenate)(string[] ["Next", "End", "--------------"], w386) -> (w377:string[])
                            n148 = call "Search Unsorted 1D Array.vim"("element"=w376, "unsorted 1D array"=w377) -> ("index of element"=w374:i32)  [unwired: 9 in]
                            n149 = Greater Or Equal To 0?(x=w374) -> (x >= 0?=w375:bool)
                            n150 = control-ref of="stepsRing"() -> (w394:refnum<vi>)
                            n151 = Select(t=w374, s=w375, f=0) -> (s? t:f=w373:i32)
                            n152 = property on="stepName" class="Str"("Visible"=FALSE) -> ()  [unwired: 2 in, 2 out]
                            n153 = property on="Property Node" class="Ring (strict)"(reference=w394, error in=w395, "Position"=w393, "RingText.Size"=w390, "RingText.Font"=w392, "Visible"=w388, "Key Focus"=w388, "Strings []"=w377, "Disabled Items []"=i32[] [2], "Value"=w373) -> (error out=w384:errorcluster)  [unwired: 1 out]
                          }
                          frame 4 {
                            n154 = property on="stepsRing" class="Ring (strict)"(error in=w401, "Visible"=FALSE) -> (error out=w399:errorcluster)  [unwired: 1 in, 1 out]
                            n155 = property on="stepName" class="Str"(error in=w399, "Visible"=FALSE) -> (error out=w398:errorcluster)  [unwired: 1 in, 1 out]
                          }
                        }
                      }
                    }
                  }
                }
                n156 = Enqueue Element(queue=w323, element="System: Event User Handler") -> (queue out=w322:refnum<queue>)  [unwired: 2 in, 2 out]
              }
              event "stepName": Value Change {
                w407 = 0  # Step column
                n157 = event-data() -> ("NewVal"=w410:string)  [unwired: 1 in]
                n158 = local read "Cell Position"() -> (w409:T2)
                n159 = property on="Sequence List" class="MCListbox (strict)"() -> (error out=w412:errorcluster, "ItemNames"=w413:string[][])  [unwired: 2 in, 1 out]
                n160 = Unbundle(w409) -> ("Row"=w408:i32)  [unwired: 1 out]
                n161 = Replace Array Subset(array=w413, new element=w410, index (row)=w408, index (col)=w407) -> (w406:string[][])
                n162 = property on="Sequence List" class="MCListbox (strict)"(error in=w412, "ItemNames"=w406) -> (error out=w411:errorcluster)  [unwired: 1 in, 1 out]
                n163 = Enqueue Element(queue=w404, element="System: Event User Handler") -> (queue out=w405:refnum<queue>)  [unwired: 2 in, 2 out]
              }
              event "stepsRing": Value Change {
                n164 = event-data() -> ("CtlRef"=w420:refnum<vi>, "NewVal"=w418:u16)  [unwired: 1 in]
                n165 = property class="Ring (strict)"(reference=w420) -> (error out=w416:errorcluster, "Strings []"=w419:string[])  [unwired: 1 in, 1 out]
                n166 = Index Array(array=w419, index=w418) -> (element=w417:string)
                n167 = property on="Sequence List" class="MCListbox (strict)"(error in=w416) -> (error out=w429:errorcluster, "ItemNames"=w430:string[][])  [unwired: 1 in, 1 out]
                n168 = local read "Cell Position"() -> (w427:T2)
                n169 = Unbundle(w427) -> ("Row"=w422:i32, "Column"=w421:i32)
                n170 = Replace Array Subset(array=w430, new element=w417, index (row)=w422, index (col)=w421) -> (w426:string[][])
                n171 = property on="Sequence List" class="MCListbox (strict)"(error in=w429, "ItemNames"=w426) -> (error out=w428:errorcluster)  [unwired: 1 in, 1 out]
                n172 = Enqueue Element(queue=w424, element="System: Event User Handler") -> (queue out=w425:refnum<queue>)  [unwired: 2 in, 2 out]
              }
              event Timeout {
                n173 = event-data() -> ()  [unwired: 1 in, 3 out]
              }
            }
          }
          frame "System:Start" {
            # "Exec Mode\n1.) RUN -- Call by main program to run production\n2.) DEBUG -- VI Run it self in TOP level\n3.) OPEN VI -- Open front panel and block diagram of subVI\n4.) EDIT -- Run VI with allow user to edit criteria ,and sequence"
            # "If not run top level then use execMode from configure"
            # "Do not modify"
            n174 = control-ref of="This VI"() -> (w447:refnum<vi>)
            n175 = property class="VI"(reference=w447) -> (error out=w451:errorcluster, "Exec.State"=w453:T13)  [unwired: 1 in, 1 out]
            n176 = Unbundle By Name(w438) -> ("testConfigCluster.execMode"=w444:T9)
            n177 = Equal?(x=T13."Run top level", y=w453) -> (x = y?=w446:bool)
            n178 = local write "Tab Control"(enum32{"Sequence", "Input", "Output"}."Sequence" ("Tab Control")) -> ()
            n179 = Not(x=w446) -> (.not. x?=w445:bool)
            n180 = Select(t=w444, s=w445, f=__TEST__STEP__VAR__UI__EXEC__MODE__."Debug") -> (s? t:f=w437:T9)
            n181 = Bundle By Name(cluster=w438, "testConfigCluster.execMode"=w437) -> (w439:T4)
            n182 = case shown="\"Run\"" w437 {
              tunnel: w451 -> [_ _]
              tunnel: w450 -> [w457 w466]
              tunnel: [w456 w465] -> w449
              tunnel: w442 -> [w455 w464]
              tunnel: [w455 w464] -> w441
              tunnel: [w454 w463] -> w440
              tunnel: w439 -> [w454 w463]
              frame "Run" {
                n183 = for {
                  tunnel: w457 -> [w461]
                  tunnel: [w460] -> w456
                  tunnel: string[] ["System: Initialize", "System: Initial UI", "System: Load sequence config file", "System: Begin-Process"] -> [w459] mode=indexing
                  n184 = Enqueue Element(queue=w461, element=w459) -> (queue out=w460:refnum<queue>)  [unwired: 2 in, 2 out]
                }
              }
              frame Default {
                n185 = for {
                  tunnel: w466 -> [w469]
                  tunnel: [w468] -> w465
                  tunnel: string[] ["System: Initialize", "System: Initial UI", "System: Load sequence config file", "System: Event User Handler"] -> [w467] mode=indexing
                  n186 = Enqueue Element(queue=w469, element=w467) -> (queue out=w468:refnum<queue>)  [unwired: 2 in, 2 out]
                }
              }
            }
          }
          frame "System: Initialize" {
            # "Do not modify"
            n187 = Unbundle By Name(w472) -> ("testConfigCluster.execMode"=w471:T9)
            n188 = case shown="\"Run\"" w471 {
              tunnel: w472 -> [w476 w482]
              tunnel: [w476 w481] -> w475
              frame "Run" {
                # "Only \"Run\" mode will use reference control from VI who called this sequence module"
              }
              frame Default {
                n189 = control-ref of="testTable"() -> (w480:refnum<vi>)
                n190 = control-ref of="displayMsg"() -> (w479:refnum<vi>)
                n191 = local write "disMsg"(w479) -> ()
                n192 = local read "criteriaINI"() -> (w477:path)
                n193 = Bundle By Name(cluster=w482, "testConfigCluster.execMode"=__TEST__STEP__VAR__UI__EXEC__MODE__."Debug", "testConfigCluster.userControls.testTable"=w480, "testConfigCluster.userControls.dialog"=w479, "testConfigCluster.criteriaINI"=w477) -> (w481:T4)
              }
            }
          }
          frame "System: Initial UI" {
            w489 = 0 ("currentItem")
            # "Display criteria file path"
            # "Do not modify"
            n194 = Unbundle By Name(w484) -> ("testConfigCluster.execMode"=w492:T9)
            n195 = Unbundle By Name(w484) -> ("testConfigCluster.criteriaINI"=w485:path)
            n196 = property on="stepsRing" class="Ring (strict)"("Visible"=FALSE) -> (error out=w488:errorcluster)  [unwired: 2 in, 1 out]
            n197 = local write "currenIndex"(w489) -> ()
            n198 = local write "currentRetest"(w489) -> ()
            n199 = local write "totalSeqIndex"(w489) -> ()
            n200 = local write "criteriaINI"(w485) -> ()
            n201 = property on="stepName" class="Str"(error in=w488, "Visible"=FALSE) -> ()  [unwired: 1 in, 2 out]
            n202 = case shown="Default" w492 {
              tunnel: w484 -> [w502 w515]
              tunnel: [w497 w512] -> w494
              tunnel: [w502 w515] -> w493
              tunnel: w491 -> [w496 w507]
              tunnel: [w496 w507] -> w490
              frame "Run" {
                n203 = control-ref of="exitButton"() -> (w500:refnum<vi>)
                n204 = control-ref of="saveButton"() -> (w499:refnum<vi>)
                n205 = control-ref of="runButton"() -> (w498:refnum<vi>)
                n206 = Build Array(w500, w499, w498) -> (w501:refnum<vi>[])
                n207 = for {
                  tunnel: w501 -> [w505] mode=indexing
                  tunnel: [w504] -> w497
                  w503 = FALSE ("Value")
                  n208 = property class="Bool (strict)"(reference=w505, "Visible"=w503, "Value"=w503) -> (error out=w504:errorcluster)  [unwired: 1 in, 1 out]
                }
              }
              frame Default {
                n209 = Unbundle By Name(w515) -> ("testConfigCluster.userControls.dialog"=w514:refnum<vi>, "testConfigCluster"=w516:T8)
                n210 = Unbundle By Name(w515) -> ("stepData"=w518:T5)
                n211 = control-ref of="exitButton"() -> (w510:refnum<vi>)
                n212 = control-ref of="saveButton"() -> (w509:refnum<vi>)
                n213 = control-ref of="runButton"() -> (w508:refnum<vi>)
                n214 = Build Array(w510, w509, w508) -> (w511:refnum<vi>[])
                n215 = for {
                  tunnel: w511 -> [w525] mode=indexing
                  tunnel: [w523] -> w506
                  n216 = property class="Bool (strict)"(reference=w525, "Visible"=TRUE ("Value"), "Value"=FALSE) -> (error out=w523:errorcluster)  [unwired: 1 in, 1 out]
                }
                n217 = call <userlib>:"Tool.Update_Result_To_Table.vi"("Action"=__TABLE__ACTION__."Initial", "testConfigCluster"=w516, "error in (no error)"=w506, "seqDataIn"=w518) -> ("error out"=w520:errorcluster, "stepDutPara(Out)"=w517:T5)  [unwired: 6 in]
                n218 = call <userlib>:"Tool.Update_Result_To_Table.vi"("Action"=__TABLE__ACTION__."Clear", "testConfigCluster"=w516, "error in (no error)"=w520, "seqDataIn"=w517) -> ("error out"=w513:errorcluster)  [unwired: 6 in, 1 out]
                n219 = invoke class="Str" method="Reinit To Default"(reference=w514, error in=w513) -> (error out=w512:errorcluster)  [unwired: 1 in, 2 out]
              }
            }
          }
          frame "System: Load sequence config file" {
            # "Do not modify"
            n220 = control-ref of="This VI"() -> (w534:refnum<vi>)
            n221 = property class="VI"(reference=w534) -> ("Path"=w530:path)  [unwired: 1 in, 2 out]
            n222 = call <userlib>:"Get_variable_json_&_seq_csv_paths.vi"("seqPath"=w530) -> ("errorOut"=w528:errorcluster, "FoundAll ?"=w527:bool, "var&seqPaths[]"=w529:path[])  [unwired: 7 in, 1 out]
            n223 = for {
              shift-right: [w548] -> w533
              shift-left: w528 -> [w550]
              shift-right: [w544] -> w531
              shift-left: w532 -> [w545]
              tunnel: w529 -> [w543] mode=indexing
              tunnel: w527 -> [w539]
              n224 = call <vilib>:"Check if File or Folder Exists.vi"("error in (no error)"=w550, "path"=w543) -> ("error out"=w547:errorcluster, "file or folder exists?"=w541:bool, "dup path"=w538:path)  [unwired: 7 in]
              n225 = Empty String/Path?(string/path=w538) -> (empty?=w549:bool)
              n226 = Strip Path(path=w538) -> (name=w537:string)  [unwired: 1 out]
              n227 = Not(x=w549) -> (.not. x?=w542:bool)
              n228 = call <vilib>:"Clear Errors.vi"("error in (no error)"=w547) -> ("error out"=w546:errorcluster)  [unwired: 5 in, 1 out]
              n229 = Compound Arithmetic op=AND(w539, w542, w541) -> (w540:bool)
              n230 = case shown="\"sequence.csv\"" w537 {
                tunnel: w546 -> [w556 w587]
                tunnel: w538 -> [w553 w584]
                tunnel: [w555 w586] -> w548
                tunnel: w540 -> [w554 w585]
                tunnel: w545 -> [w552 w583]
                tunnel: [w551 w583] -> w544
                frame "variable.json", Default {
                  n231 = case shown="True" w554 {
                    tunnel: w556 -> [w558 w578]
                    tunnel: [w567 w573] -> w555
                    tunnel: w553 -> [w566 w571]
                    tunnel: w552 -> [w557 w570]
                    tunnel: [w557 w569] -> w551
                    frame False {
                      n232 = local read "userDef"() -> (w565:T3)
                      n233 = call <vilib>:"Flatten To JSON String.vi"("error in (no error)"=w558, "Variant"=w565) -> ("error out"=w559:errorcluster, "JSON String"=w560:string)  [unwired: 8 in]
                      n234 = Open/Create/Replace File(file path (use dialog)=w566, error in=w559, operation (0:open)=T10."create") -> (refnum out=w564:refnum<file>, error out=w562:errorcluster)  [unwired: 3 in, 1 out]
                      n235 = Write to Text File(file (use dialog)=w564, text=w560, error in=w562) -> (refnum out=w563:refnum<file>, error out=w561:errorcluster)  [unwired: 1 in, 1 out]
                      n236 = Close File(refnum=w563, error in=w561) -> (error out=w567:errorcluster)  [unwired: 1 out]
                    }
                    frame True {
                      n237 = Open/Create/Replace File(file path (use dialog)=w571, error in=w578, operation (0:open)=T10."open") -> (refnum out=w580:refnum<file>, error out=w582:errorcluster)  [unwired: 3 in, 1 out]
                      n238 = Read from Text File(file (use dialog)=w580, error in=w582) -> (refnum out=w579:refnum<file>, text=w575:string, error out=w581:errorcluster)  [unwired: 2 in, 1 out]
                      n239 = Close File(refnum=w579, error in=w581) -> (error out=w576:errorcluster)  [unwired: 1 out]
                      n240 = call <vilib>:"Unflatten From JSON String.vi"("Type and Defaults"=w570, "error in (no error)"=w576, "JSON String"=w575) -> ("error out"=w574:errorcluster, "Variant"=w572:variant)  [unwired: 7 in]
                      n241 = Variant To Data(error in=w574, type=w570, Variant=w572) -> (data=w569:T3, error out=w573:errorcluster)
                      n242 = local write "userDef"(w569) -> ()
                    }
                  }
                  n243 = local write "varFilePath"(w553) -> ()
                }
                frame "sequence.csv" {
                  n244 = case shown="True" w585 {
                    tunnel: w587 -> [w593 w608]
                    tunnel: [w591 w605] -> w586
                    tunnel: w584 -> [w588 w604]
                    frame False {
                      n245 = Open/Create/Replace File(file path (use dialog)=w588, error in=w593, operation (0:open)=T10."create") -> (refnum out=w595:refnum<file>, error out=w594:errorcluster)  [unwired: 3 in, 1 out]
                      n246 = Close File(refnum=w595, error in=w594) -> (error out=w592:errorcluster)  [unwired: 1 out]
                      n247 = property on="Sequence List" class="MCListbox (strict)"(error in=w592, "ItemNames"=string[][] [], "Value"=i32[] [] ("Sequence List")) -> (error out=w591:errorcluster)  [unwired: 1 in, 1 out]
                    }
                    frame True {
                      # "Delete first column (Enable flag)"
                      n248 = call-poly <vilib>:"Read Delimited Spreadsheet.vi"("file path (dialog if empty)"=w604, "error in (no error)"=w608, "delimiter (\\t)"="," ("delimiter (\\t)")) -> ("all rows"=w602:string[][], "error out"=w607:errorcluster)  [unwired: 7 in, 4 out]
                      n249 = Delete From Array(array=w602, index (col)=0 ("index (row)")) -> (deleted portion=w600:string[], array with subset deleted=w601:string[][])  [unwired: 2 in]
                      n250 = To Lower Case(string=w600) -> (all lower case string=w599:string[])
                      n251 = for {
                        tunnel: [w615] -> _ mode=indexing if=w612
                        tunnel: w599 -> [w614] mode=indexing
                        tunnel: [w609] -> w598 mode=indexing
                        i -> [w615]
                        n252 = Equal?(x=w614, y="enable") -> (x = y?=w612:bool)
                        n253 = Select(t=38, s=w612, f=37) -> (s? t:f=w609:i32)
                      }
                      n254 = property on="Sequence List" class="MCListbox (strict)"(error in=w607, "ItemNames"=w601, "ItemSyms"=w598, "Value"=i32[] [] ("Sequence List")) -> (error out=w605:errorcluster)  [unwired: 1 in, 1 out]
                    }
                  }
                  n255 = local write "seqFilePath"(w584) -> ()
                }
              }
            }
          }
          frame "System: Begin-Process" {
            # "Do not modify"
            n256 = property on="Sequence List" class="MCListbox (strict)"() -> ("ItemNames"=w618:string[][])  [unwired: 2 in, 2 out]
            n257 = Index Array(array=w618, index (col)=0 ("disabled index (col)")) -> (element=w621:string[])  [unwired: 1 in]
            n258 = Array Size(array=w621) -> (size(s)=w620:i32)
            n259 = local write "totalSeqIndex"(w620) -> ()
            n260 = local write "seqData[](Process)"(w618) -> ()
            n261 = local write "seqData[](Original)"(w618) -> ()
            n262 = Empty Array?(array=w618) -> (empty?=w625:bool)
            n263 = Select(t="System:End", s=w625, f="System:Pre-Process") -> (s? t:f=w626:string)
            n264 = Enqueue Element(queue=w628, element=w626) -> (queue out=w627:refnum<queue>)  [unwired: 2 in, 2 out]
          }
          frame "System:Pre-Process" {
            # "Get first index of arrays"
            # "Do not modify"
            n265 = local read "seqData[](Process)"() -> (w637:string[][])
            n266 = local read "currenIndex"() -> (w633:i32)
            n267 = Build Array(w633) -> (w635:i32[])
            n268 = Index Array(array=w637, index (row)=w633) -> (element=w636:string[])  [unwired: 1 in]
            n269 = property on="Sequence List" class="MCListbox (strict)"("Value"=w635) -> ("ItemSyms"=w634:i32[])  [unwired: 2 in, 2 out]
            n270 = Index Array(array=w634, index=w633) -> (element=w632:i32)
            n271 = Equal?(x=w632, y=38) -> (x = y?=w630:bool)
            n272 = case shown="False" w630 {
              tunnel: w642 -> [w664 w678]
              tunnel: [w663 w677] -> w641
              tunnel: [w662 w676] -> w640
              tunnel: w638 -> [w653 w673]
              tunnel: w636 -> [w651 w671]
              frame True {
                # "Clear data"
                n273 = Index Array(array=w651, index #1=T16."StepName", index #2=T16."PassTo", index #3=T16."FailTo", index #4=T16."ErrorTo", index #5=T15."Re-test") -> (element #1=w650:string, element #2=w656:string, element #3=w655:string, element #4=w654:string, element #5=w648:string)
                n274 = call <userlib>:"SEQ.Update_Seq_Var_Module.Init.vi"("mainVar"=w653) -> ("mainVarOut"=w661:T4)  [unwired: 2 in]
                n275 = Build Array (concatenate)(w650, string[] ["System:Post-Process:Check_Retest", "System:Post-Process:Update_Result"]) -> (w644:string[])
                n276 = Decimal String To Number(string=w648, default (0L)=u8 0 ("default (0 I32)")) -> (number=w647:u8)  [unwired: 1 in, 1 out]
                n277 = Reverse 1D Array(array=w644) -> (reversed array=w643:string[])
                n278 = Get Date/Time In Seconds() -> (seconds since 1Jan1904=w652:timestamp)
                n279 = for {
                  tunnel: w664 -> [w667]
                  tunnel: [w666] -> w663
                  tunnel: w643 -> [w665] mode=indexing
                  n280 = Enqueue Element At Opposite End(queue=w667, element=w665) -> (queue out=w666:refnum<queue>)  [unwired: 2 in, 2 out]
                }
                n281 = Bundle By Name(cluster=w661, "stepData.stepName"=w650, "stepData.passTo"=w656, "stepData.failTo"=w655, "stepData.errorTo"=w654, "stepData.retest"=w647, "stepData.startTime"=w652) -> (w662:T4)
              }
              frame False {
                # "Clear data"
                n282 = Index Array(array=w671, index=T16."StepName") -> (element=w670:string)
                n283 = call <userlib>:"SEQ.Update_Seq_Var_Module.Init.vi"("mainVar"=w673) -> ("mainVarOut"=w675:T4)  [unwired: 2 in]
                n284 = Get Date/Time In Seconds() -> (seconds since 1Jan1904=w672:timestamp)
                n285 = Bundle By Name(cluster=w675, "stepData.stepName"=w670, "stepData.startTime"=w672, "stepData.statusType"=__STEP__DATA__STATUS__TYPE__."SKIPPED") -> (w676:T4)
                n286 = Enqueue Element(queue=w678, element="System:Post-Process:Update_Result") -> (queue out=w677:refnum<queue>)  [unwired: 2 in, 2 out]
              }
            }
          }
          frame "System:Post-Process:Check_Retest" {
            # "Do not modify"
            n287 = Unbundle By Name(w683) -> ("stepData.statusType"=w684:T7)
            n288 = case shown="\"FAIL\"" w684 {
              tunnel: w683 -> [w689 w704]
              tunnel: [w688 w704] -> w682
              tunnel: w681 -> [w690 w703]
              tunnel: [w687 w703] -> w680
              frame "FAIL" {
                # "Retest over limit or have no Retest"
                n289 = Unbundle By Name(w689) -> ("stepData.retest"=w691:u8)
                n290 = local read "currentRetest"() -> (w692:u8)
                n291 = Greater Or Equal?(x=w692, y=w691) -> (x >= y?=w686:bool)
                n292 = case shown="False" w686 {
                  tunnel: w690 -> [w699 w701]
                  tunnel: w689 -> [w695 w702]
                  tunnel: [w695 w702] -> w688
                  tunnel: [w697 w701] -> w687
                  frame False {
                    # "Retest again"
                    n293 = local read "currentRetest"() -> (w694:u8)
                    n294 = Flush Queue(queue=w699) -> (queue out=w698:refnum<queue>)  [unwired: 1 in, 2 out]
                    n295 = Increment(x=w694) -> (x+1=w693:u8)
                    n296 = local write "currentRetest"(w693) -> ()
                    n297 = Enqueue Element(queue=w698, element="System:Pre-Process") -> (queue out=w697:refnum<queue>)  [unwired: 2 in, 2 out]
                  }
                  frame True {
                    # "Clear"
                    n298 = local write "currentRetest"(u8 0 ("currentItem")) -> ()
                  }
                }
              }
              frame Default {
              }
            }
          }
          frame "System:Post-Process:Update_Result" {
            # "Do not modify"
            n299 = Unbundle By Name(w707) -> ("stepData.statusType"=w708:T7)
            n300 = case shown="\"DONE\", \"PASS\"" w708 {
              tunnel: w707 -> [w718 w720 w722 _]
              tunnel: [w717 w719 w721 ""] -> w709
              frame "DONE", "PASS" {
                n301 = Unbundle By Name(w718) -> ("stepData.passTo"=w717:string)
              }
              frame "FAIL" {
                n302 = Unbundle By Name(w720) -> ("stepData.failTo"=w719:string)
              }
              frame "ERROR" {
                n303 = Unbundle By Name(w722) -> ("stepData.errorTo"=w721:string)
              }
              frame Default {
              }
            }
            n304 = local write "Tab Control"(enum32{"Sequence", "Input", "Output"}."Output" ("Tab Control")) -> ()
            n305 = local read "seqData[](Process)"() -> (w712:string[][])
            n306 = local read "currenIndex"() -> (w711:i32)
            n307 = call <userlib>:"ATMF.Get_Seq_Value_Index.vi"("seqData[]"=w712, "stepData.GoTo"=w709, "currenIndex"=w711) -> ("newIndex"=w710:i32)  [unwired: 8 in]
            n308 = call <userlib>:"SEQ.Append_Test_Result_To_Table.vi"("seqDataIn"=w707) -> ("seqDataOut"=w715:T4)  [unwired: 8 in, 2 out]
            n309 = case shown="-2" w710 {
              selector: w710 -> [w724 _ _]
              tunnel: w714 -> [w731 w734 w737]
              tunnel: [w730 w733 w736] -> w713
              frame Default {
                # "If new index more than total index size then finish testing"
                n310 = local read "totalSeqIndex"() -> (w726:i32)
                n311 = local write "currenIndex"(w724) -> ()
                n312 = Greater Or Equal?(x=w724, y=w726) -> (x >= y?=w725:bool)
                n313 = Select(t="System:End" ("element"), s=w725, f="System:Pre-Process" ("element")) -> (s? t:f=w727:string)
                n314 = Enqueue Element(queue=w731, element=w727) -> (queue out=w730:refnum<queue>)  [unwired: 2 in, 2 out]
              }
              frame -1 {
                # "Cannot find searched step name\n\nGo to end seq"
                n315 = Enqueue Element(queue=w734, element="System:End") -> (queue out=w733:refnum<queue>)  [unwired: 2 in, 2 out]
              }
              frame -2 {
                # "Go to end"
                n316 = Enqueue Element(queue=w737, element="System:End") -> (queue out=w736:refnum<queue>)  [unwired: 2 in, 2 out]
              }
            }
          }
          frame "System:End" {
            # "Do not modify"
            n317 = Unbundle By Name(w740) -> ("testConfigCluster.execMode"=w739:T9)
            n318 = case shown="Default" w739 {
              tunnel: [FALSE TRUE] -> w746
              tunnel: w745 -> [w752 w755]
              tunnel: [w752 w755] -> w744
              tunnel: w740 -> [w751 w754]
              tunnel: [w751 w754] -> w743
              tunnel: w742 -> [w748 w753]
              tunnel: [w749 w753] -> w741
              frame Default {
                n319 = Enqueue Element(queue=w748, element="System: Event User Handler") -> (queue out=w749:refnum<queue>)  [unwired: 2 in, 2 out]
              }
              frame "Run" {
              }
            }
          }
          frame Default {
            # "Do not modify"
            n320 = Concatenate Strings("Default case --> " ("message"), w763, "\nPlease check your test case is valid" ("string")) -> (w760:string)
            n321 = call "Display Message to User2"("Enable"=TRUE, "Message"=w760) -> ("error out"=w759:errorcluster)  [unwired: 8 in, 1 out]
          }
          frame "------------Developer Case------------" {
            # "Do not modify"
          }
          frame "init" {
            w775 = T19[] [enum."FCT_FAN_SW", enum."DMM_SW", enum."USB_Reset"] items=["Reset", "APOS_SENSE", "ANEG_SENSE", "DPOS_SENSE", "FCT_SW1", "FCT_SW2", "FCT_SW3", "ANEG_LOAD", "APOS_LOAD", "DPOS_LOAD", "Short ANEG", "Short APOS", "Short DPOS", "meas_PSU_1_12V", "meas_PSU_2_12V", "meas_PSU_3_12V", "meas_UUT_APOS_voltage", "meas_UUT_ANEG_voltage", "meas_UUT_DPOS_voltage", "meas_LOAD_APOS_voltage", "meas_LOAD_ANEG_voltage", "meas_LOAD_DPOS_voltage", "UUT_FCT_power_SW", "Burn_in_FAN_SW", "FCT_FAN_SW", "FCT_24V_SW", "USB_Reset", "DMM_SW"]
            w788 = refnum<visa-resource-name> refnum ("VISA resource name")
            n322 = call "Read Ini.vi"("error in (no error)"=w790, "key"="DMM3058", "section"="Instrument") -> ("error out"=w789:errorcluster, "value"=w791:string)  [unwired: 7 in]
            n323 = call "Read Array Ini.vi"("error in (no error)"=w789, "Read_key"=string[] ["IO_Card", "Diagnostic_board"], "Section"="IO Card") -> ("error out"=w801:errorcluster, "Result_Value"=w800:string[])  [unwired: 7 in]
            n324 = call <userlib>:"SEQ.Update_Seq_Var_Module.Step_Name.vi"("Decription"="init", "mainVar"=w812, "Step Name"=w780) -> ("mainVarOut"=w808:T4)  [unwired: 4 in]
            n325 = call "Read Array Ini.vi"("error in (no error)"=w801, "Read_key"=string[] ["Control_BOX_LED", "UUT_LED", "Diagnostic_board"], "Section"="LED_left") -> ("error out"=w776:errorcluster, "Result_Value"=w798:string[])  [unwired: 7 in]
            n326 = Index Array(array=w800) -> (element #1=w799:string)  [unwired: 2 in, 1 out]
            n327 = Index Array(array=w798) -> (element #1=w797:string, element #2=w796:string, element #3=w773:string)  [unwired: 3 in]
            n328 = Type Cast(type=w788, x=w796) -> (*(type *) &x=w794:refnum<visa-resource-name>)
            n329 = Type Cast(type=w788, x=w797) -> (*(type *) &x=w795:refnum<visa-resource-name>)
            n330 = Type Cast(type=w788, x=w773) -> (*(type *) &x=w777:refnum<visa-resource-name>)
            n331 = Type Cast(type=w788, x=w791) -> (*(type *) &x=w782:refnum<visa-resource-name>)
            n332 = Type Cast(type=w788, x=w799) -> (*(type *) &x=w774:refnum<visa-resource-name>)
            n333 = call "DM3058 drive.vi"("Function Choose"=DM3058_Function_Choose."Init", "error in (no error)"=w776, "VISA resource name"=w782) -> ("error out"=w785:errorcluster, "VISA resource name out"=w786:refnum<visa-resource-name>)  [unwired: 6 in, 1 out]
            n334 = Bundle By Name(cluster=w806, "DMM3058"=w782, "IO_Card"=w774, "Diagnostic_board"=w777, "Control_BOX_LED"=w795, "UUT_LED"=w794) -> (w781:T1)
            n335 = call "DM3058 drive.vi"("Function Choose"=DM3058_Function_Choose."Config", "error in (no error)"=w785, "parameter"=T17 {"Reset (True)"=TRUE, "ID Query (True)"=FALSE, "Auto Range (T:Enable)"=FALSE, "Function (0: DC Volts)"=0, "Range Select"=enum."20V", "Absolute Resolution (0: 5.5 Rate:Slow)"=1}, "VISA resource name"=w786) -> ("error out"=w778:errorcluster)  [unwired: 5 in, 2 out]
            n336 = for {
              tunnel: w778 -> [w818]
              tunnel: w774 -> [w817]
              tunnel: [w815] -> w772
              tunnel: w775 -> [w814] mode=indexing
              n337 = call "DCDC_Command.vi"("error in (no error)"=w818, "State"=TRUE, "Function Choose"=w814, "VISA resource in"=w817) -> ("error out"=w815:errorcluster)  [unwired: 4 in, 3 out]
            }
            n338 = call-poly <userlib>:"[Polymorphic] SEQ.Update_Seq_Var_Module.vi"("UUT Error"=w772, "System Error In"=w779, "seqDataIn"=w808) -> ("System Error Out"=w810:errorcluster, "seqDataOut"=w811:T4)  [unwired: 7 in]
          }
          frame "Power On" {
            n339 = Unbundle By Name(w835) -> ("IO_Card"=w823:refnum<visa-resource-name>)
            n340 = call <userlib>:"SEQ.Update_Seq_Var_Module.Step_Name.vi"("Decription"="Power On", "mainVar"=w842, "Step Name"=w829) -> ("mainVarOut"=w826:T4)  [unwired: 4 in]
            n341 = call "DCDC_Command.vi"("error in (no error)"=w827, "State"=TRUE, "Function Choose"=DCDC_Command."UUT_FCT_power_SW", "VISA resource in"=w823) -> ("error out"=w825:errorcluster, "VISA resource out"=w822:refnum<visa-resource-name>)  [unwired: 4 in, 2 out]
            n342 = call "Stall Data Flow.vim"("value in"=w825, "milliseconds to wait"=u32 2000) -> ("value out"=w820:errorcluster)  [unwired: 1 out]
            n343 = call "DCDC_Command.vi"("error in (no error)"=w820, "State"=FALSE, "Function Choose"=DCDC_Command."USB_Reset", "VISA resource in"=w822) -> ("error out"=w821:errorcluster)  [unwired: 4 in, 3 out]
            n344 = Format Into String(format string="%s    ", w829) -> (resulting string=w832:string)  [unwired: 2 in, 1 out]
            n345 = local read "disMsg"() -> (w833:refnum<vi>)
            n346 = call <userlib>:"ATMF.Disaplay_Msg_Console.vi"("errorIn"=w821, "Message"=w832, "dialogIn"=w833) -> ("errorOut"=w830:errorcluster)  [unwired: 7 in, 1 out]
            n347 = call-poly <userlib>:"[Polymorphic] SEQ.Update_Seq_Var_Module.vi"("UUT Error"=w830, "System Error In"=w828, "seqDataIn"=w826) -> ("System Error Out"=w840:errorcluster, "seqDataOut"=w841:T4)  [unwired: 7 in]
          }
          frame "Measure VPS1" {
            w857 = DCDC_Command."meas_PSU_1_12V" ("Function Choose")
            n348 = Unbundle By Name(w858) -> ("DMM3058"=w847:refnum<visa-resource-name>, "IO_Card"=w844:refnum<visa-resource-name>)
            n349 = call "DCDC_Command.vi"("error in (no error)"=w846, "State"=TRUE, "Function Choose"=w857, "VISA resource in"=w844) -> ("error out"=w848:errorcluster, "VISA resource out"=w860:refnum<visa-resource-name>)  [unwired: 4 in, 2 out]
            n350 = call <userlib>:"SEQ.Update_Seq_Var_Module.Step_Name.vi"("Decription"="Measure VPS1", "mainVar"=w874, "Step Name"=w851) -> ("mainVarOut"=w870:T4)  [unwired: 4 in]
            n351 = Unbundle By Name(w868) -> ("VSP1 Max"=w867:dbl, "VSP1 Min"=w865:dbl)
            n352 = call "DM3058 drive.vi"("Function Choose"=DM3058_Function_Choose."Measure", "error in (no error)"=w848, "VISA resource name"=w847) -> ("error out"=w861:errorcluster, "Measurement"=w850:dbl)  [unwired: 6 in, 1 out]
            n353 = Number To Fractional String(number=w867) -> (F-format string=w866:string)  [unwired: 3 in]
            n354 = Number To Fractional String(number=w865) -> (F-format string=w864:string)  [unwired: 3 in]
            n355 = call-poly <userlib>:"[Polymorphic] SEQ.Update_Seq_Var_Module.Set_Max_Min.vi"("stepData.min"=w864, "stepData.max"=w866, "seqDataIn"=w870) -> ("seqDataOut"=w869:T4)  [unwired: 8 in]
            n356 = Format Into String(format string="%s    %d", w851, w850) -> (resulting string=w855:string)  [unwired: 2 in, 1 out]
            n357 = call "DCDC_Command.vi"("error in (no error)"=w861, "State"=FALSE, "Function Choose"=w857, "VISA resource in"=w860) -> ("error out"=w852:errorcluster)  [unwired: 4 in, 3 out]
            n358 = local read "disMsg"() -> (w856:refnum<vi>)
            n359 = call <userlib>:"ATMF.Disaplay_Msg_Console.vi"("errorIn"=w852, "Message"=w855, "dialogIn"=w856) -> ("errorOut"=w853:errorcluster)  [unwired: 7 in, 1 out]
            n360 = call-poly <userlib>:"[Polymorphic] SEQ.Update_Seq_Var_Module.vi"("UUT Error"=w853, "System Error In"=w849, "value"=w850, "Unit"="V", "seqDataIn"=w869) -> ("System Error Out"=w872:errorcluster, "seqDataOut"=w873:T4)  [unwired: 5 in]
          }
          frame "Measure VPS2" {
            w884 = DCDC_Command."meas_PSU_2_12V" ("Function Choose")
            n361 = Unbundle By Name(w887) -> ("DMM3058"=w885:refnum<visa-resource-name>, "IO_Card"=w886:refnum<visa-resource-name>)
            n362 = call "DCDC_Command.vi"("error in (no error)"=w888, "State"=TRUE, "Function Choose"=w884, "VISA resource in"=w886) -> ("error out"=w889:errorcluster, "VISA resource out"=w891:refnum<visa-resource-name>)  [unwired: 4 in, 2 out]
            n363 = call <userlib>:"SEQ.Update_Seq_Var_Module.Step_Name.vi"("Decription"="Measure VPS2", "mainVar"=w906, "Step Name"=w878) -> ("mainVarOut"=w902:T4)  [unwired: 4 in]
            n364 = Unbundle By Name(w900) -> ("VSP2 Max"=w899:dbl, "VSP2 Min"=w897:dbl)
            n365 = call "DM3058 drive.vi"("Function Choose"=DM3058_Function_Choose."Measure", "error in (no error)"=w889, "VISA resource name"=w885) -> ("error out"=w892:errorcluster, "Measurement"=w877:dbl)  [unwired: 6 in, 1 out]
            n366 = Number To Fractional String(number=w899) -> (F-format string=w898:string)  [unwired: 3 in]
            n367 = Number To Fractional String(number=w897) -> (F-format string=w896:string)  [unwired: 3 in]
            n368 = call-poly <userlib>:"[Polymorphic] SEQ.Update_Seq_Var_Module.Set_Max_Min.vi"("stepData.min"=w896, "stepData.max"=w898, "seqDataIn"=w902) -> ("seqDataOut"=w901:T4)  [unwired: 8 in]
            n369 = Format Into String(format string="%s    %d", w878, w877) -> (resulting string=w882:string)  [unwired: 2 in, 1 out]
            n370 = local read "disMsg"() -> (w883:refnum<vi>)
            n371 = call "DCDC_Command.vi"("error in (no error)"=w892, "State"=FALSE, "Function Choose"=w884, "VISA resource in"=w891) -> ("error out"=w879:errorcluster)  [unwired: 4 in, 3 out]
            n372 = call <userlib>:"ATMF.Disaplay_Msg_Console.vi"("errorIn"=w879, "Message"=w882, "dialogIn"=w883) -> ("errorOut"=w880:errorcluster)  [unwired: 7 in, 1 out]
            n373 = call-poly <userlib>:"[Polymorphic] SEQ.Update_Seq_Var_Module.vi"("UUT Error"=w880, "System Error In"=w876, "value"=w877, "Unit"="V", "seqDataIn"=w901) -> ("System Error Out"=w904:errorcluster, "seqDataOut"=w905:T4)  [unwired: 5 in]
          }
          frame "Measure VPS3" {
            w916 = DCDC_Command."meas_PSU_3_12V" ("Function Choose")
            n374 = Unbundle By Name(w917) -> ("DMM3058"=w919:refnum<visa-resource-name>, "IO_Card"=w920:refnum<visa-resource-name>)
            n375 = call "DCDC_Command.vi"("error in (no error)"=w918, "State"=TRUE, "Function Choose"=w916, "VISA resource in"=w920) -> ("error out"=w921:errorcluster, "VISA resource out"=w923:refnum<visa-resource-name>)  [unwired: 4 in, 2 out]
            n376 = call <userlib>:"SEQ.Update_Seq_Var_Module.Step_Name.vi"("Decription"="Measure VPS3", "mainVar"=w938, "Step Name"=w909) -> ("mainVarOut"=w934:T4)  [unwired: 4 in]
            n377 = Unbundle By Name(w932) -> ("VSP3 Max"=w931:dbl, "VSP3 Min"=w929:dbl)
            n378 = call "DM3058 drive.vi"("Function Choose"=DM3058_Function_Choose."Measure", "error in (no error)"=w921, "VISA resource name"=w919) -> ("error out"=w924:errorcluster, "Measurement"=w910:dbl)  [unwired: 6 in, 1 out]
            n379 = Number To Fractional String(number=w931) -> (F-format string=w930:string)  [unwired: 3 in]
            n380 = Number To Fractional String(number=w929) -> (F-format string=w928:string)  [unwired: 3 in]
            n381 = call-poly <userlib>:"[Polymorphic] SEQ.Update_Seq_Var_Module.Set_Max_Min.vi"("stepData.min"=w928, "stepData.max"=w930, "seqDataIn"=w934) -> ("seqDataOut"=w933:T4)  [unwired: 8 in]
            n382 = Format Into String(format string="%s    %d", w909, w910) -> (resulting string=w914:string)  [unwired: 2 in, 1 out]
            n383 = local read "disMsg"() -> (w915:refnum<vi>)
            n384 = call "DCDC_Command.vi"("error in (no error)"=w924, "State"=FALSE, "Function Choose"=w916, "VISA resource in"=w923) -> ("error out"=w911:errorcluster)  [unwired: 4 in, 3 out]
            n385 = call <userlib>:"ATMF.Disaplay_Msg_Console.vi"("errorIn"=w911, "Message"=w914, "dialogIn"=w915) -> ("errorOut"=w912:errorcluster)  [unwired: 7 in, 1 out]
            n386 = call-poly <userlib>:"[Polymorphic] SEQ.Update_Seq_Var_Module.vi"("UUT Error"=w912, "System Error In"=w908, "value"=w910, "Unit"="V", "seqDataIn"=w933) -> ("System Error Out"=w936:errorcluster, "seqDataOut"=w937:T4)  [unwired: 5 in]
          }
          frame "Measure L1 ON" {
            n387 = Unbundle By Name(w946) -> ("Control_BOX_LED"=w956:refnum<visa-resource-name>)
            n388 = call <userlib>:"SEQ.Update_Seq_Var_Module.Step_Name.vi"("Decription"="Measure L1 ON", "mainVar"=w961, "Step Name"=w950) -> ("mainVarOut"=w957:T4)  [unwired: 4 in]
            n389 = Unbundle By Name(w945) -> ()  [unwired: 2 out]
            n390 = call "LED_Command.vi"("L lower limit"=25, "Hue lower limit"=65, "L upper limit"=70, "Hue upper limit"=150, "error in (no error)"=w949, "channel"="1", "VISA resource in"=w956) -> ("error out"=w948:errorcluster, "Result"=w944:bool)  [unwired: 1 in, 2 out]
            n391 = Format Into String(format string="%s    %s", w950, w944) -> (resulting string=w954:string)  [unwired: 2 in, 1 out]
            n392 = local read "disMsg"() -> (w955:refnum<vi>)
            n393 = call <userlib>:"ATMF.Disaplay_Msg_Console.vi"("errorIn"=w948, "Message"=w954, "dialogIn"=w955) -> ("errorOut"=w952:errorcluster)  [unwired: 7 in, 1 out]
            n394 = call-poly <userlib>:"[Polymorphic] SEQ.Update_Seq_Var_Module.vi"("UUT Error"=w952, "System Error In"=w951, "value"=w944, "seqDataIn"=w957) -> ("System Error Out"=w959:errorcluster, "seqDataOut"=w960:T4)  [unwired: 6 in]
          }
          frame "Measure L3 ON" {
            n395 = Unbundle By Name(w979) -> ("Control_BOX_LED"=w978:refnum<visa-resource-name>)
            n396 = call <userlib>:"SEQ.Update_Seq_Var_Module.Step_Name.vi"("Decription"="Measure L3 ON", "mainVar"=w984, "Step Name"=w971) -> ("mainVarOut"=w980:T4)  [unwired: 4 in]
            n397 = Unbundle By Name(w968) -> ()  [unwired: 2 out]
            n398 = call "LED_Command.vi"("L lower limit"=25, "Hue lower limit"=65, "L upper limit"=70, "Hue upper limit"=150, "error in (no error)"=w977, "channel"="3", "VISA resource in"=w978) -> ("error out"=w970:errorcluster, "Result"=w967:bool)  [unwired: 1 in, 2 out]
            n399 = Format Into String(format string="%s    %s", w971, w967) -> (resulting string=w974:string)  [unwired: 2 in, 1 out]
            n400 = local read "disMsg"() -> (w975:refnum<vi>)
            n401 = call <userlib>:"ATMF.Disaplay_Msg_Console.vi"("errorIn"=w970, "Message"=w974, "dialogIn"=w975) -> ("errorOut"=w972:errorcluster)  [unwired: 7 in, 1 out]
            n402 = call-poly <userlib>:"[Polymorphic] SEQ.Update_Seq_Var_Module.vi"("UUT Error"=w972, "System Error In"=w976, "value"=w967, "seqDataIn"=w980) -> ("System Error Out"=w982:errorcluster, "seqDataOut"=w983:T4)  [unwired: 6 in]
          }
          frame "Measure UUT D3 ON" {
            n403 = Unbundle By Name(w1002) -> ("UUT_LED"=w1001:refnum<visa-resource-name>)
            n404 = call <userlib>:"SEQ.Update_Seq_Var_Module.Step_Name.vi"("Decription"=" Measure UUT D3 ON ", "mainVar"=w1007, "Step Name"=w995) -> ("mainVarOut"=w1003:T4)  [unwired: 4 in]
            n405 = Unbundle By Name(w991) -> ()  [unwired: 2 out]
            n406 = call "LED_Command.vi"("L lower limit"=25, "Hue lower limit"=65, "L upper limit"=70, "Hue upper limit"=150, "error in (no error)"=w1000, "channel"="1", "VISA resource in"=w1001) -> ("error out"=w992:errorcluster, "Result"=w990:bool)  [unwired: 1 in, 2 out]
            n407 = Format Into String(format string="%s    %s", w995, w990) -> (resulting string=w998:string)  [unwired: 2 in, 1 out]
            n408 = local read "disMsg"() -> (w999:refnum<vi>)
            n409 = call <userlib>:"ATMF.Disaplay_Msg_Console.vi"("errorIn"=w992, "Message"=w998, "dialogIn"=w999) -> ("errorOut"=w996:errorcluster)  [unwired: 7 in, 1 out]
            n410 = call-poly <userlib>:"[Polymorphic] SEQ.Update_Seq_Var_Module.vi"("UUT Error"=w996, "System Error In"=w994, "value"=w990, "seqDataIn"=w1003) -> ("System Error Out"=w1005:errorcluster, "seqDataOut"=w1006:T4)  [unwired: 6 in]
          }
          frame "Measure UUT D5 ON" {
            n411 = Unbundle By Name(w1025) -> ("UUT_LED"=w1024:refnum<visa-resource-name>)
            n412 = call <userlib>:"SEQ.Update_Seq_Var_Module.Step_Name.vi"("Decription"="Measure UUT D5 ON", "mainVar"=w1030, "Step Name"=w1017) -> ("mainVarOut"=w1026:T4)  [unwired: 4 in]
            n413 = Unbundle By Name(w1014) -> ()  [unwired: 2 out]
            n414 = call "LED_Command.vi"("L lower limit"=25, "Hue lower limit"=65, "L upper limit"=70, "Hue upper limit"=150, "error in (no error)"=w1023, "channel"="3", "VISA resource in"=w1024) -> ("error out"=w1016:errorcluster, "Result"=w1013:bool)  [unwired: 1 in, 2 out]
            n415 = Format Into String(format string="%s    %s", w1017, w1013) -> (resulting string=w1020:string)  [unwired: 2 in, 1 out]
            n416 = local read "disMsg"() -> (w1021:refnum<vi>)
            n417 = call <userlib>:"ATMF.Disaplay_Msg_Console.vi"("errorIn"=w1016, "Message"=w1020, "dialogIn"=w1021) -> ("errorOut"=w1018:errorcluster)  [unwired: 7 in, 1 out]
            n418 = call-poly <userlib>:"[Polymorphic] SEQ.Update_Seq_Var_Module.vi"("UUT Error"=w1018, "System Error In"=w1022, "value"=w1013, "seqDataIn"=w1026) -> ("System Error Out"=w1028:errorcluster, "seqDataOut"=w1029:T4)  [unwired: 6 in]
          }
          frame "Measure UUT D6 ON" {
            n419 = Unbundle By Name(w1048) -> ("UUT_LED"=w1047:refnum<visa-resource-name>)
            n420 = call <userlib>:"SEQ.Update_Seq_Var_Module.Step_Name.vi"("Decription"="Measure UUT D6 ON", "mainVar"=w1053, "Step Name"=w1040) -> ("mainVarOut"=w1049:T4)  [unwired: 4 in]
            n421 = Unbundle By Name(w1037) -> ()  [unwired: 2 out]
            n422 = call "LED_Command.vi"("L lower limit"=25, "Hue lower limit"=65, "L upper limit"=70, "Hue upper limit"=150, "error in (no error)"=w1046, "channel"="4", "VISA resource in"=w1047) -> ("error out"=w1039:errorcluster, "Result"=w1036:bool)  [unwired: 1 in, 2 out]
            n423 = Format Into String(format string="%s    %s", w1040, w1036) -> (resulting string=w1043:string)  [unwired: 2 in, 1 out]
            n424 = local read "disMsg"() -> (w1044:refnum<vi>)
            n425 = call <userlib>:"ATMF.Disaplay_Msg_Console.vi"("errorIn"=w1039, "Message"=w1043, "dialogIn"=w1044) -> ("errorOut"=w1041:errorcluster)  [unwired: 7 in, 1 out]
            n426 = call-poly <userlib>:"[Polymorphic] SEQ.Update_Seq_Var_Module.vi"("UUT Error"=w1041, "System Error In"=w1045, "value"=w1036, "seqDataIn"=w1049) -> ("System Error Out"=w1051:errorcluster, "seqDataOut"=w1052:T4)  [unwired: 6 in]
          }
          frame "Measure UUT D8 ON" {
            n427 = Unbundle By Name(w1071) -> ("UUT_LED"=w1070:refnum<visa-resource-name>)
            n428 = call <userlib>:"SEQ.Update_Seq_Var_Module.Step_Name.vi"("Decription"="Measure UUT D8 ON", "mainVar"=w1076, "Step Name"=w1065) -> ("mainVarOut"=w1072:T4)  [unwired: 4 in]
            n429 = Unbundle By Name(w1060) -> ()  [unwired: 2 out]
            n430 = call "LED_Command.vi"("L lower limit"=25, "Hue lower limit"=65, "L upper limit"=70, "Hue upper limit"=150, "error in (no error)"=w1063, "channel"="6", "VISA resource in"=w1070) -> ("error out"=w1062:errorcluster, "Result"=w1059:bool)  [unwired: 1 in, 2 out]
            n431 = Format Into String(format string="%s    %s", w1065, w1059) -> (resulting string=w1068:string)  [unwired: 2 in, 1 out]
            n432 = local read "disMsg"() -> (w1069:refnum<vi>)
            n433 = call <userlib>:"ATMF.Disaplay_Msg_Console.vi"("errorIn"=w1062, "Message"=w1068, "dialogIn"=w1069) -> ("errorOut"=w1066:errorcluster)  [unwired: 7 in, 1 out]
            n434 = call-poly <userlib>:"[Polymorphic] SEQ.Update_Seq_Var_Module.vi"("UUT Error"=w1066, "System Error In"=w1064, "value"=w1059, "seqDataIn"=w1072) -> ("System Error Out"=w1074:errorcluster, "seqDataOut"=w1075:T4)  [unwired: 6 in]
          }
          frame "Measure APOS UUT Voltages" {
            n435 = Unbundle By Name(w1098) -> ("DMM3058"=w1095:refnum<visa-resource-name>, "IO_Card"=w1097:refnum<visa-resource-name>, "Diagnostic_board"=w1080:refnum<visa-resource-name>)
            n436 = call <userlib>:"SEQ.Update_Seq_Var_Module.Step_Name.vi"("Decription"=" Measure APOS UUT Voltages", "mainVar"=w1102, "Step Name"=w1088) -> ("mainVarOut"=w1085:T4)  [unwired: 4 in]
            n437 = Unbundle By Name(w1094) -> ("APOS Max"=w1079:dbl, "APOS Min"=w1078:dbl)
            n438 = disable-structure shown="Enabled" {
              disable-tunnel: w1097 -> [w1110 _]
              disable-tunnel: w1096 -> [w1109 w1122]
              disable-tunnel: w1095 -> [w1108 _]
              disable-tunnel: [w1105 w1121] -> w1089
              disable-tunnel: [w1104 _] -> _
              disable-tunnel: [_ w1120] -> w1081
              disable-tunnel: w1080 -> [_ w1119]
              disable-tunnel: w1079 -> [_ w1117]
              disable-tunnel: w1078 -> [_ w1116]
              frame Disabled {
                w1106 = DCDC_Command."meas_UUT_APOS_voltage" ("Function Choose")
                n439 = call "DCDC_Command.vi"("error in (no error)"=w1109, "State"=TRUE, "Function Choose"=w1106, "VISA resource in"=w1110) -> ("error out"=w1107:errorcluster, "VISA resource out"=w1112:refnum<visa-resource-name>)  [unwired: 4 in, 2 out]
                n440 = call "DM3058 drive.vi"("Function Choose"=DM3058_Function_Choose."Measure", "error in (no error)"=w1107, "VISA resource name"=w1108) -> ("error out"=w1111:errorcluster, "Measurement"=w1104:dbl)  [unwired: 6 in, 1 out]
                n441 = call "DCDC_Command.vi"("error in (no error)"=w1111, "State"=FALSE, "Function Choose"=w1106, "VISA resource in"=w1112) -> ("error out"=w1105:errorcluster)  [unwired: 4 in, 3 out]
              }
              frame Enabled {
                n442 = for {
                  N: 200 -> [_]
                  tunnel: [w1124] -> w1120
                  tunnel: w1119 -> [w1127]
                  shift-right: [w1128] -> w1121
                  shift-left: w1122 -> [w1129]
                  tunnel: w1117 -> [w1126]
                  tunnel: w1116 -> [w1125]
                  stop <- w1123 stop-if-true
                  n443 = call "UUT modules Read Temperature and Voltages.vi"("error in (no error)"=w1129, "VISA resource name"=w1127) -> ("error out"=w1128:errorcluster, "APOS_Voltage"=w1124:dbl)  [unwired: 3 in, 5 out]
                  n444 = In Range and Coerce(upper limit=w1126, x=w1124, lower limit=w1125) -> (In Range?=w1123:bool)  [unwired: 1 out]
                }
              }
            }
            n445 = Number To Fractional String(number=w1079) -> (F-format string=w1087:string)  [unwired: 3 in]
            n446 = Number To Fractional String(number=w1078) -> (F-format string=w1086:string)  [unwired: 3 in]
            n447 = call-poly <userlib>:"[Polymorphic] SEQ.Update_Seq_Var_Module.Set_Max_Min.vi"("stepData.min"=w1086, "stepData.max"=w1087, "seqDataIn"=w1085) -> ("seqDataOut"=w1084:T4)  [unwired: 8 in]
            n448 = Format Into String(format string="%s    %d", w1088, w1081) -> (resulting string=w1092:string)  [unwired: 2 in, 1 out]
            n449 = local read "disMsg"() -> (w1093:refnum<vi>)
            n450 = call <userlib>:"ATMF.Disaplay_Msg_Console.vi"("errorIn"=w1089, "Message"=w1092, "dialogIn"=w1093) -> ("errorOut"=w1090:errorcluster)  [unwired: 7 in, 1 out]
            n451 = call-poly <userlib>:"[Polymorphic] SEQ.Update_Seq_Var_Module.vi"("UUT Error"=w1090, "System Error In"=w1083, "value"=w1081, "Unit"="V", "seqDataIn"=w1084) -> ("System Error Out"=w1100:errorcluster, "seqDataOut"=w1099:T4)  [unwired: 5 in]
          }
          frame "Measure ANEG UUT Voltages" {
            n452 = Unbundle By Name(w1148) -> ("DMM3058"=w1149:refnum<visa-resource-name>, "IO_Card"=w1150:refnum<visa-resource-name>, "Diagnostic_board"=w1132:refnum<visa-resource-name>)
            n453 = call <userlib>:"SEQ.Update_Seq_Var_Module.Step_Name.vi"("Decription"="Measure ANEG UUT Voltages", "mainVar"=w1154, "Step Name"=w1141) -> ("mainVarOut"=w1137:T4)  [unwired: 4 in]
            n454 = Unbundle By Name(w1147) -> ("ANEG Max"=w1131:dbl, "ANEG Min"=w1130:dbl)
            n455 = disable-structure shown="Enabled" {
              disable-tunnel: w1150 -> [w1162 _]
              disable-tunnel: w1149 -> [w1161 _]
              disable-tunnel: [w1157 w1173] -> w1142
              disable-tunnel: [w1156 _] -> _
              disable-tunnel: w1134 -> [_ w1174]
              disable-tunnel: [_ w1172] -> w1133
              disable-tunnel: w1132 -> [_ w1171]
              disable-tunnel: w1131 -> [_ w1169]
              disable-tunnel: w1130 -> [_ w1168]
              frame Disabled {
                w1158 = DCDC_Command."meas_UUT_ANEG_voltage" ("Function Choose")
                n456 = call "DCDC_Command.vi"("State"=TRUE, "Function Choose"=w1158, "VISA resource in"=w1162) -> ("error out"=w1160:errorcluster, "VISA resource out"=w1164:refnum<visa-resource-name>, "error in (no error)"=w1159:errorcluster)  [unwired: 4 in, 2 out]
                n457 = call "DM3058 drive.vi"("Function Choose"=DM3058_Function_Choose."Measure", "error in (no error)"=w1160, "VISA resource name"=w1161) -> ("error out"=w1163:errorcluster, "Measurement"=w1156:dbl)  [unwired: 6 in, 1 out]
                n458 = call "DCDC_Command.vi"("error in (no error)"=w1163, "State"=FALSE, "Function Choose"=w1158, "VISA resource in"=w1164) -> ("error out"=w1157:errorcluster)  [unwired: 4 in, 3 out]
              }
              frame Enabled {
                n459 = for {
                  N: 200 -> [_]
                  tunnel: [w1175] -> w1172
                  tunnel: w1171 -> [w1179]
                  shift-right: [w1180] -> w1173
                  shift-left: w1174 -> [w1181]
                  tunnel: w1169 -> [w1177]
                  tunnel: w1168 -> [w1176]
                  stop <- w1178 stop-if-true
                  n460 = call "UUT modules Read Temperature and Voltages.vi"("error in (no error)"=w1181, "VISA resource name"=w1179) -> ("error out"=w1180:errorcluster, "ANEG_Voltage"=w1175:dbl)  [unwired: 3 in, 5 out]
                  n461 = In Range and Coerce(upper limit=w1177, x=w1175, lower limit=w1176) -> (In Range?=w1178:bool)  [unwired: 1 out]
                }
              }
            }
            n462 = Number To Fractional String(number=w1131) -> (F-format string=w1139:string)  [unwired: 3 in]
            n463 = Number To Fractional String(number=w1130) -> (F-format string=w1138:string)  [unwired: 3 in]
            n464 = call-poly <userlib>:"[Polymorphic] SEQ.Update_Seq_Var_Module.Set_Max_Min.vi"("stepData.min"=w1138, "stepData.max"=w1139, "seqDataIn"=w1137) -> ("seqDataOut"=w1136:T4)  [unwired: 8 in]
            n465 = Format Into String(format string="%s    %d", w1141, w1133) -> (resulting string=w1145:string)  [unwired: 2 in, 1 out]
            n466 = local read "disMsg"() -> (w1146:refnum<vi>)
            n467 = call <userlib>:"ATMF.Disaplay_Msg_Console.vi"("errorIn"=w1142, "Message"=w1145, "dialogIn"=w1146) -> ("errorOut"=w1143:errorcluster)  [unwired: 7 in, 1 out]
            n468 = call-poly <userlib>:"[Polymorphic] SEQ.Update_Seq_Var_Module.vi"("UUT Error"=w1143, "System Error In"=w1140, "value"=w1133, "Unit"="V", "seqDataIn"=w1136) -> ("System Error Out"=w1152:errorcluster, "seqDataOut"=w1151:T4)  [unwired: 5 in]
          }
          frame "Measure DPOS UUT Voltages" {
            n469 = Unbundle By Name(w1200) -> ("DMM3058"=w1199:refnum<visa-resource-name>, "IO_Card"=w1201:refnum<visa-resource-name>, "Diagnostic_board"=w1184:refnum<visa-resource-name>)
            n470 = call <userlib>:"SEQ.Update_Seq_Var_Module.Step_Name.vi"("Decription"=" Measure DPOS UUT Voltages", "mainVar"=w1206, "Step Name"=w1191) -> ("mainVarOut"=w1188:T4)  [unwired: 4 in]
            n471 = Unbundle By Name(w1198) -> ("DPOS Max"=w1183:dbl, "DPOS Min"=w1182:dbl)
            n472 = disable-structure shown="Enabled" {
              disable-tunnel: w1202 -> [w1212 w1226]
              disable-tunnel: w1201 -> [w1211 _]
              disable-tunnel: w1199 -> [w1210 _]
              disable-tunnel: [w1209 w1225] -> w1194
              disable-tunnel: [w1208 w1224] -> w1185
              disable-tunnel: w1184 -> [_ w1223]
              disable-tunnel: w1183 -> [_ w1221]
              disable-tunnel: w1182 -> [_ w1220]
              frame Disabled {
                w1213 = DCDC_Command."meas_UUT_APOS_voltage" ("Function Choose")
                n473 = call "DCDC_Command.vi"("error in (no error)"=w1212, "State"=TRUE, "Function Choose"=w1213, "VISA resource in"=w1211) -> ("error out"=w1214:errorcluster, "VISA resource out"=w1216:refnum<visa-resource-name>)  [unwired: 4 in, 2 out]
                n474 = call "DM3058 drive.vi"("Function Choose"=DM3058_Function_Choose."Measure", "error in (no error)"=w1214, "VISA resource name"=w1210) -> ("error out"=w1215:errorcluster, "Measurement"=w1208:dbl)  [unwired: 6 in, 1 out]
                n475 = call "DCDC_Command.vi"("error in (no error)"=w1215, "State"=FALSE, "Function Choose"=w1213, "VISA resource in"=w1216) -> ("error out"=w1209:errorcluster)  [unwired: 4 in, 3 out]
              }
              frame Enabled {
                n476 = for {
                  N: 200 -> [_]
                  tunnel: [w1228] -> w1224
                  tunnel: w1223 -> [w1231]
                  shift-right: [w1232] -> w1225
                  shift-left: w1226 -> [w1233]
                  tunnel: w1221 -> [w1230]
                  tunnel: w1220 -> [w1229]
                  stop <- w1227 stop-if-true
                  n477 = call "UUT modules Read Temperature and Voltages.vi"("error in (no error)"=w1233, "VISA resource name"=w1231) -> ("error out"=w1232:errorcluster, "DPOS_Voltage"=w1228:dbl)  [unwired: 3 in, 5 out]
                  n478 = In Range and Coerce(upper limit=w1230, x=w1228, lower limit=w1229) -> (In Range?=w1227:bool)  [unwired: 1 out]
                }
              }
            }
            n479 = Number To Fractional String(number=w1183) -> (F-format string=w1190:string)  [unwired: 3 in]
            n480 = Number To Fractional String(number=w1182) -> (F-format string=w1189:string)  [unwired: 3 in]
            n481 = call-poly <userlib>:"[Polymorphic] SEQ.Update_Seq_Var_Module.Set_Max_Min.vi"("stepData.min"=w1189, "stepData.max"=w1190, "seqDataIn"=w1188) -> ("seqDataOut"=w1187:T4)  [unwired: 8 in]
            n482 = Format Into String(format string="%s    %d", w1191, w1185) -> (resulting string=w1196:string)  [unwired: 2 in, 1 out]
            n483 = local read "disMsg"() -> (w1197:refnum<vi>)
            n484 = call <userlib>:"ATMF.Disaplay_Msg_Console.vi"("errorIn"=w1194, "Message"=w1196, "dialogIn"=w1197) -> ("errorOut"=w1195:errorcluster)  [unwired: 7 in, 1 out]
            n485 = call-poly <userlib>:"[Polymorphic] SEQ.Update_Seq_Var_Module.vi"("UUT Error"=w1195, "System Error In"=w1193, "value"=w1185, "Unit"="V", "seqDataIn"=w1187) -> ("System Error Out"=w1204:errorcluster, "seqDataOut"=w1203:T4)  [unwired: 5 in]
          }
          frame "Clean" {
            n486 = call <userlib>:"SEQ.Update_Seq_Var_Module.Step_Name.vi"("Decription"="Clean", "mainVar"=w1239, "Step Name"=w1240) -> ("mainVarOut"=w1241:T4)  [unwired: 4 in]
            n487 = call-poly <userlib>:"[Polymorphic] SEQ.Update_Seq_Var_Module.vi"("System Error In"=w1237, "seqDataIn"=w1241) -> ("System Error Out"=w1235:errorcluster, "seqDataOut"=w1234:T4)  [unwired: 8 in]
          }
        }
      }
      frame Error {
        # "Bypass system error out to main program"
        n488 = Flush Queue(queue=w1247) -> (queue out=w1249:refnum<queue>)  [unwired: 1 in, 2 out]
        n489 = Enqueue Element(queue=w1249, element="End") -> (queue out=w1250:refnum<queue>)  [unwired: 2 in, 2 out]
      }
    }
    n490 = call <userlib>:"SEQ.Post_Process.CheckSeqDone&StopEvent.vi"("sysErrorIn(noError)"=w26, "mainVar"=w28) -> ("sysErrorIOut"=w25:errorcluster, "userStop??"=w24:bool, "mainVarOut"=w27:T4)  [unwired: 7 in]
    n491 = Or(x=w24, y=w23) -> (x .or. y?=w22:bool)
  }
  "System Error Out" <- w11
  n492 = Unbundle By Name(w5) -> ("testConfigCluster"=w4:T8)
  n493 = Flush Queue(queue=w16) -> (queue out=w18:refnum<queue>, error out=w12:errorcluster)  [unwired: 1 in, 1 out]
  n494 = Release Queue(queue=w18, error in (no error)=w12) -> (error out=w13:errorcluster)  [unwired: 1 in, 2 out]
  n495 = call <vilib>:"Clear Errors.vi"("error in (no error)"=w13) -> ()  [unwired: 5 in, 2 out]
  n496 = To Variant(anything=w4) -> (Variant=→"variantOut":variant)
